vi "Create_Trajectory_Using_TrajectoryLibrary_ORIG.vi"() -> ()   [LabVIEW 2019]
doc: "This utility creates trajectories based on the robot configuration, constraints and defined waypoints."
uses:
  <vilib>/Rock Robotics/WPI/ThirdParty/JAS_Junk/TrajLib/Trajectory_Library.lvlib
  <vilib>/Utility/xml.llb/Write to XML File(string).vi
  <vilib>/Rock Robotics/WPI/ThirdParty/JAS_Junk/TrajLib/TRANSLATION2D.ctl
  <vilib>/Rock Robotics/WPI/ThirdParty/JAS_Junk/TrajLib/ROTATION2D.ctl
  <vilib>/Rock Robotics/WPI/ThirdParty/JAS_Junk/TrajLib/POSE2D.ctl
  <vilib>/Rock Robotics/WPI/ThirdParty/JAS_Junk/TrajLib/TRAJ_STATE.ctl
  <vilib>/Rock Robotics/WPI/ThirdParty/JAS_Junk/TrajLib/TRAJECTORY.ctl
  <vilib>/Utility/xml.llb/Read From XML File(string).vi
  <vilib>/Rock Robotics/WPI/ThirdParty/JAS_Junk/TrajLib/DISPLAY_WEIGHTED_WAYPOINT.ctl
  <vilib>/Rock Robotics/WPI/ThirdParty/JAS_Junk/TrajLib/DIFF_DRIVE_KINEMATICS.ctl
  <vilib>/Rock Robotics/WPI/ThirdParty/JAS_Junk/TrajLib/TRAJ_CONSTRAINT_DIIF_DRIVE_KINEMATICS.ctl
  <vilib>/Rock Robotics/WPI/ThirdParty/JAS_Junk/TrajLib/TRAJ_CONSTRAINT_CENTRIPETAL_ACCEL.ctl
  <vilib>/Analysis/Matrix/Datatypes/RealMatrix.ctl
  <vilib>/Analysis/Matrix/NI_Matrix.lvlib
  <vilib>/Rock Robotics/WPI/ThirdParty/JAS_Junk/TrajLib/SWERVE_DRIVE_KINEMATICS.ctl
  <vilib>/Rock Robotics/WPI/ThirdParty/JAS_Junk/TrajLib/TRAJ_CONSTRAINT_SWERVE_DRIVE_KINEMATICS.ctl
  <vilib>/Rock Robotics/WPI/ThirdParty/JAS_Junk/TrajLib/SIMPLE_MOTOR_FF.ctl
  <vilib>/Rock Robotics/WPI/ThirdParty/JAS_Junk/TrajLib/TRAJ_CONSTRAINT_DIIF_DRIVE_VOLTAGE.ctl
  <vilib>/Rock Robotics/WPI/ThirdParty/JAS_Junk/TrajLib/MECA_DRIVE_KINEMATICS.ctl
  <vilib>/Rock Robotics/WPI/ThirdParty/JAS_Junk/TrajLib/TRAJ_CONSTRAINT_MECA_DRIVE_KINEMATICS.ctl
  <vilib>/Rock Robotics/WPI/ThirdParty/JAS_Junk/TrajLib/TRAJ_CONFIG.ctl
  TrajCreateUnitsENUM.ctl
  TrajCreateConfig_V3.ctl
panel:
  in  "End Program":bool
  in  "Tab Control":T1(tab)
  out "Config File Read\nWithout Error":bool
  out "Config File  Read Error":errorcluster
  out "Read Config File Comment":string
  in  "Read Config File Name":path
  in  "ReadConfigFile":bool
  in  "Field Selector":string(combo)
  in  "Units Selector":T2
  in  "MaxVelocity":dbl=50.0 format="%17.1f"
  in  "MaxAcceleration":dbl=40.0 format="%17.1f"
  out "MaxVelocity M/S":dbl=2.0 format="%17.4f"
  out "MaxAcceleration M/S^2":dbl=1.3 format="%17.4f"
  in  "Right Rear":T3={"X"=-0.5, "Y"=0.5} {"Y" format="%14.3f"; "X" format="%14.3f"}
  in  "Left Rear":T3={"X"=-0.5, "Y"=-0.5} {"Y" format="%14.3f"; "X" format="%14.3f"}
  in  "Right Front":T3={"X"=0.5, "Y"=0.5} {"Y" format="%14.3f"; "X" format="%14.3f"}
  in  "Left Front":T3={"X"=0.5, "Y"=-0.5} {"Y" format="%14.3f"; "X" format="%14.3f"}
  in  "Use Centripetal\nAcceleration\nConstaint":bool=TRUE
  out "Max Cent Accel M/S^2":dbl=1.0 format="%20.4f"
  in  "Max Cent Accel":dbl=20.0 format="%20.1f"
  in  "Use Diff Drive\nKinematic\nConstraint":bool=TRUE
  out "Wheelbase Width M":dbl=0.66 format="%20.4f"
  in  "Wheelbase Width":dbl=20.866 format="%20.1f"
  in  "Max Voltage":dbl=12.0 format="%20.4f"
  in  "SIMPLE_MOTOR_FF":T4={"Ks"=0.9, "Kv"=0.22199, "Ka"=0.04876} {"Ka" format="%13.4f"; "Kv" format="%13.4f"; "Ks" format="%13.4f"}
  in  "Use Diff Drive\nVoltage\nConstraint":bool=TRUE
  in  "Wheels":T3[](array[typedef])=[{"X"=0.5, "Y"=-0.5}, {"X"=0.5, "Y"=0.5}, {"X"=-0.5, "Y"=0.5}, {"X"=-0.5, "Y"=-0.5}] {"Y" format="%14.3f"; "X" format="%14.3f"}
  in  "Use Swerve Drive\nKinematics\nConstraint":bool
  in  "Use Mecanum \nDrive Kinematics\nConstraint":bool
  out "Left Front M":T3 {"Y" format="%14.3f"; "X" format="%14.3f"}
  out "Right Front M":T3 {"Y" format="%14.3f"; "X" format="%14.3f"}
  out "Left Rear M":T3 {"Y" format="%14.3f"; "X" format="%14.3f"}
  out "Right Rear M":T3 {"Y" format="%14.3f"; "X" format="%14.3f"}
  out "SIMPLE_MOTOR_FF M":T4 {"Ka" format="%13.4f"; "Kv" format="%13.4f"; "Ks" format="%13.4f"}
  out "Wheels M":T3[](array[typedef]) {"Y" format="%14.3f"; "X" format="%14.3f"}
  in  "WayPoints":T5[](array[typedef])=[{"X"=15.0, "Y"=105.0, "ANGLE"=-45.0, "WEIGHT"=12.0}, {"X"=105.0, "Y"=65.0, "ANGLE"=0.0, "WEIGHT"=12.0}, {"X"=210.0, "Y"=106.0, "ANGLE"=45.0, "WEIGHT"=12.0}, {"X"=350.0, "Y"=105.0, "ANGLE"=-45.0, "WEIGHT"=12.0}] {"WEIGHT" format="%13.3f"; "ANGLE" format="%13.3f"; "Y" format="%13.3f"; "X" format="%13.3f"}
  in  "Spline Type":enum32{"Radio Selection 1", "Radio Selection 2"}(radio)
  in  "Reverse":bool
  in  "UseWeights":bool
  in  "Calculate\nTrajectory":bool
  out "Trajectory\nCompleted\nError Free":bool
  out "Trajectory calculation error":errorcluster
  out "Position":cluster{dbl[], dbl[]}[](graph)
  out "Field Display":T6(plugin-control)
  out "Trajectory Data":cluster{dbl[], dbl[]}[](graph)
  out "differential \ndrive \nmax speed":dbl format="%15.1f"
  out "Traj States\nSize":i32
  out "Trajectory States":T7[](array[typedef]) {"POSE"."ROTATION"."SIN" format="%13.4f"; "POSE"."ROTATION"."COS" format="%13.4f"; "POSE"."ROTATION"."VALUE" format="%13.4f"; "POSE"."TRANSLATION"."Y" format="%14.3f"; "POSE"."TRANSLATION"."X" format="%14.3f"}
  in  "Trajectory JSON File Name":path
  out "JSON File Saved\nWithout Error":bool
  out "Write CSV File Error":errorcluster
  in  "PathWeaver Length Units":T10(radio)
  in  "WriteJSONFile":bool
  out "CSV File Saved\nWithout Error":bool
  in  "Trajectory Type":enum32{"Radio Selection 1", "Radio Selection 2"}(radio)
  out "Write Trajectory\nFile Error":errorcluster
  in  "Trajectory File Comment":string
  in  "Trajectory CSV File Name":path
  in  "WriteTrajFile":bool
  out "Config File Saved\nWithout Error":bool
  out "Write Config FIle Error":errorcluster
  in  "Write Config File Comment":string
  in  "Write Config File Name":path
  in  "WriteConfigFile":bool
  # "Create Trajectory  (Use LabVIEW trajectory library)"
  # "Instructions:  \n----------------\n\nThis utility will create a trajectory, show the data on the various tabs, and optionally write a \"field absolute\" or \"robot relative\" trajectory to a file. \nTo use this utility:\n\n1) Read all of these instructions!\n2) Define the robot's physical data on the \"Robot Data\" tab.  \n3) Define the robot's movement constraints on the \"Constraints\" page.  \n4) Define the trajectory on the \"Define/Create Trajectory\" tab.  These are the beginning and ending positions/headings, and internal positions/headings.  \n    Cubic splines only use the first and last \"angle\".  The other internal \"angles\" are calculated.  Quintic splines use all the defined angles.\n5) Press the \"Calculate Trajectory\".  If a good trajectory was calculated it will be displayed.  If no errors are generated the Trajectory Complete\n    light will be on.  Errors will be displayed in the error indicator.  The path can be recalculated many times before performing any other action.\n\nAfter a Trajectory has been calculated, the \"trajectory can be written to a file.  The absolute path is converted to a robot relative trajectory.  To do this:\n1) Enter a comment to be included in the file.  Anything can be entered.\n2) Select the file name.\n3) Press \"Create Trajectory File\"  If an error occurs it will be displayed in the File Creation Error indicator.\n\nNotes:\n--------\n- All the robot parameters, path, and field dimensions are in UNITS, and DEGREES.  Select UNITS from the \"Robot Data\" page.  The resulting  \n  trajectory is converted to METERS, and RADIANS to match the rest of this library!\n- The trajectory library is the same as the WPILIB spline and trajectory library for Java and C++.\n- 2019 playing field size - width: 26 ft 11.25 In = 323.25 in , length: 52 ft 5.25 in = 629.25 in  (I didn't verify this for the 2020 version.)"
  # "Read Trajectory Waypoints and Configuration from File"
  # "ROBOT DATA"
  # "UNITS/SEC"
  # "Meters/SEC"
  # "UNITS/SEC^2"
  # "Meters/SEC^2"
  # "Simulated robot max speed is: 68.266 Inches/Second"
  # "UTILITY CONFIGURATION"
  # "Diff Kinematics Constraint"
  # "Centripetal Accel Constraint"
  # "Diff Voltage Constraint"
  # "UNITS"
  # "UNITS/SEC^2"
  # "VOLTS"
  # "METERS"
  # "METERS/SEC^2"
  # "Distance is:\nUNITS"
  # "Simulated robot wheelbase is 20.87 in"
  # "Ks = Volts\nKv = VoltSec/Meter\nKa = Volt(Sec^2)/Meter"
  # "Swerve Kinematics Constraint"
  # "Mechanum Kinematics Constraint"
  # "Values\nare \nUNITS"
  # "Values\nare \nUNITS"
  # "TRAJECTORY DEFINITION"
  # "To delete array elements or the entire array, right click on the array or element, select Data Operations, then select the action to be performed."
  # "UNITS, UNITS, DEGREES, SCALAR"
  # "INCHES/SEC"
  # "Write Trajectory to File   -   CSV, and / or JSON"
  # "Write Trajectory Waypoints and Configuration to File"
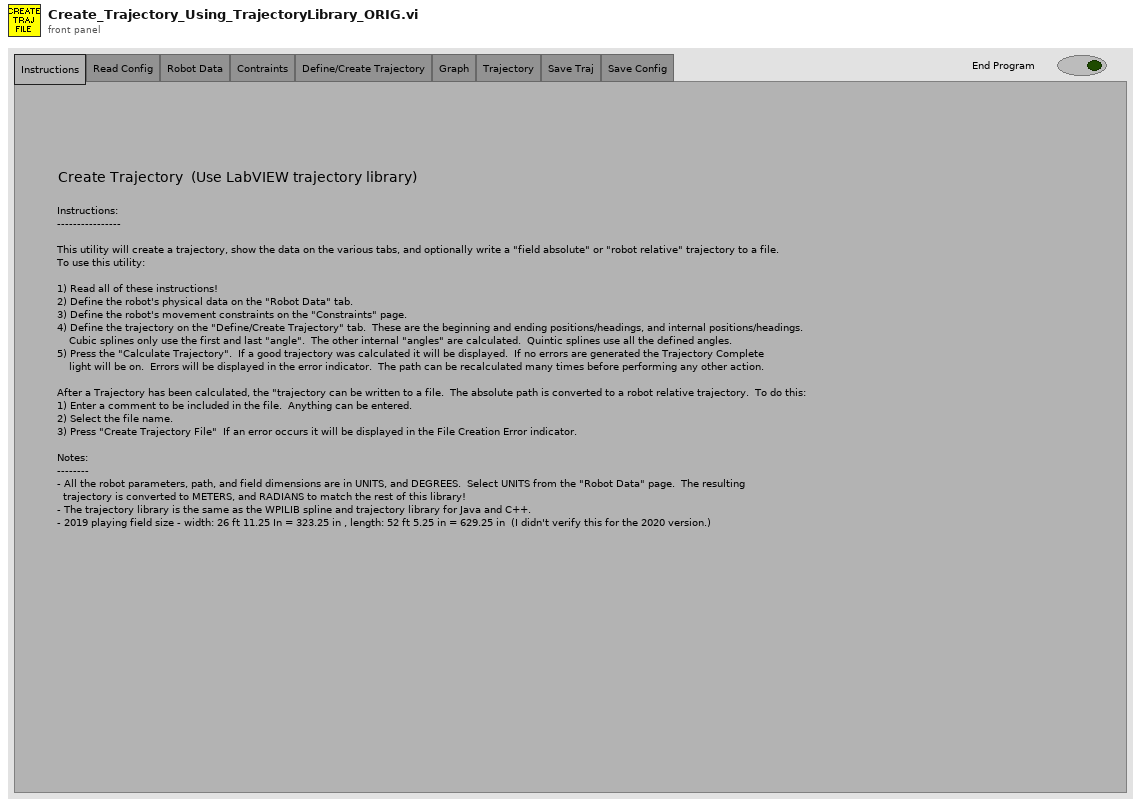
[diagram p1: front panel]
types:
  T1 = enum32{"Instructions", "Read Config", "Robot Data", "Contraints", "Define/Create Trajectory", "Graph", "Trajectory", "Save Traj", "Save Config"}
  T2 = typedef "TrajCreateUnitsENUM.ctl" = enum16{"Inches", "Feet", "Centimeters", "Meters"}
  T3 = typedef "Trajectory_Library.lvlib/TRANSLATION2D.ctl" = cluster{"X":dbl, "Y":dbl}
  T4 = typedef "Trajectory_Library.lvlib/SIMPLE_MOTOR_FF.ctl" = cluster{"Ks":dbl, "Kv":dbl, "Ka":dbl}
  T5 = typedef "Trajectory_Library.lvlib/DISPLAY_WEIGHTED_WAYPOINT.ctl" = cluster{"X":dbl, "Y":dbl, "ANGLE":dbl, "WEIGHT":dbl}
  T6 = typedef "IMAQ Image.ctl" = refnum<image>
  T7 = typedef "Trajectory_Library.lvlib/TRAJ_STATE.ctl" = cluster{"TimeSeconds":dbl, "Velocity":dbl, "Acceleration":dbl, "POSE":T8, "Curvature":dbl}
  T8 = typedef "Trajectory_Library.lvlib/POSE2D.ctl" = cluster{"TRANSLATION":T3, "ROTATION":T9}
  T9 = typedef "Trajectory_Library.lvlib/ROTATION2D.ctl" = cluster{"VALUE":dbl, "COS":dbl, "SIN":dbl}
  T10 = enum32{"Radio Selection 1", "Radio Selection 2", "Radio Selection 3", "Radio Selection 4", "Radio Selection 5"}
  T11 = typedef "Image Type" = u32
  T12 = enum8{"Enabled", "Disabled", "Disabled and Grayed Out"}
  T13 = typedef "Trajectory_Library.lvlib/TRAJECTORY.ctl" = cluster{"TotalTImeSecs":dbl, "States":T7[]}
  T14 = typedef "TrajCreateConfig_V3.ctl" = cluster{"Write Config File Name":path, "Write Config File Comment":string, "WayPoints":T5[], "TRAJECTORY_CONFIG":T15, "IsCubic":bool, "Units Selector":T2, "UseWeights":bool}
  T15 = typedef "Trajectory_Library.lvlib/TRAJ_CONFIG.ctl" = cluster{"MaxVelocity":dbl, "Max Acceleration":dbl, "StartVelocity":dbl, "End Velocity":dbl, "Reversed":bool, "DiffDrKineConstntDefined":bool, "CentAcellConstntDefined":bool, "DiffDrVoltConstntDefined":bool, "DIFF_DRIVE_KINE_CONSTRAINT":T16, "CENTRIPETAL_ACCEL_CONSTRAINT":T18, "SwerveDrKineConstntDefined":bool, "SWERVE_DRIVE_KINE_CONSTRAINT":T19, "DIFF_DRIVE_VOLTAGE_CONSTRAINT":T22, "MECANUM_DRIVE_KINE_CONSTRAINT":T23, "MecanumDrKineConstntDefined":bool}
  T16 = typedef "Trajectory_Library.lvlib/TRAJ_CONSTRAINT_DIIF_DRIVE_KINEMATICS.ctl" = cluster{"Max Speed (M/S)":dbl, "DIFF_DRIVE_KINEMATICS":T17, "Max Accel (M/S2)":dbl}
  T17 = typedef "Trajectory_Library.lvlib/DIFF_DRIVE_KINEMATICS.ctl" = cluster{"TrackWidth_Meters":dbl}
  T18 = typedef "Trajectory_Library.lvlib/TRAJ_CONSTRAINT_CENTRIPETAL_ACCEL.ctl" = cluster{"Max Cent Accel":dbl}
  T19 = typedef "Trajectory_Library.lvlib/TRAJ_CONSTRAINT_SWERVE_DRIVE_KINEMATICS.ctl" = cluster{"Max Speed (M/S)":dbl, "SwerveKinematics":T20}
  T20 = typedef "Trajectory_Library.lvlib/SWERVE_DRIVE_KINEMATICS.ctl" = cluster{"NumModules":i32, "InverseKinematics":T21, "ForwardKinematics":T21, "Modules":T3[], "PrevCoR":T3}
  T21 = typedef "NI_Matrix.lvlib/RealMatrix.ctl" = dbl[][]
  T22 = typedef "Trajectory_Library.lvlib/TRAJ_CONSTRAINT_DIIF_DRIVE_VOLTAGE.ctl" = cluster{"Max Voltage":dbl, "DIFF_DRIVE_KINEMATICS":T17, "SIMPLE_MOTOR_FF":T4}
  T23 = typedef "Trajectory_Library.lvlib/TRAJ_CONSTRAINT_MECA_DRIVE_KINEMATICS.ctl" = cluster{"Max Speed (M/S)":dbl, "MECA_DRIVE_KINEMATICS":T24}
  T24 = typedef "Trajectory_Library.lvlib/MECA_DRIVE_KINEMATICS.ctl" = cluster{"FrontLeft":T3, "FrontRight":T3, "RearLeft":T3, "RearRight":T3, "InverseKinematics":T21, "ForwardKinematics":T21, "PrevCoR":T3}
  T25 = typedef "TrajectoryUtils_Field_Info.ctl" = cluster{"FIeld_File_Name":string, "Top_Left_X":i32, "Top_Left_Y":i32, "Bottom_Right_X":i32, "Bottom_Right_Y":i32, "Field_Size_X":dbl, "Field_Size_Y":dbl, "FIeld_Size_Units":string}
  T26 = typedef "Trajectory_Library.lvlib/WEIGHTED_WAYPOINT.ctl" = cluster{"TRANSLATION":T3, "ROTATION":T9, "SCALAR":dbl}
  T27 = typedef "Trajectory_Library.lvlib/SPLINE_CTRL_VECTOR.ctl" = cluster{"Xs":dbl[], "Ys":dbl[]}
  T28 = typedef "Trajectory_Library.lvlib/CHASSIS_SPEEDS.ctl" = cluster{"vX":dbl, "vY":dbl, "vOmega":dbl}
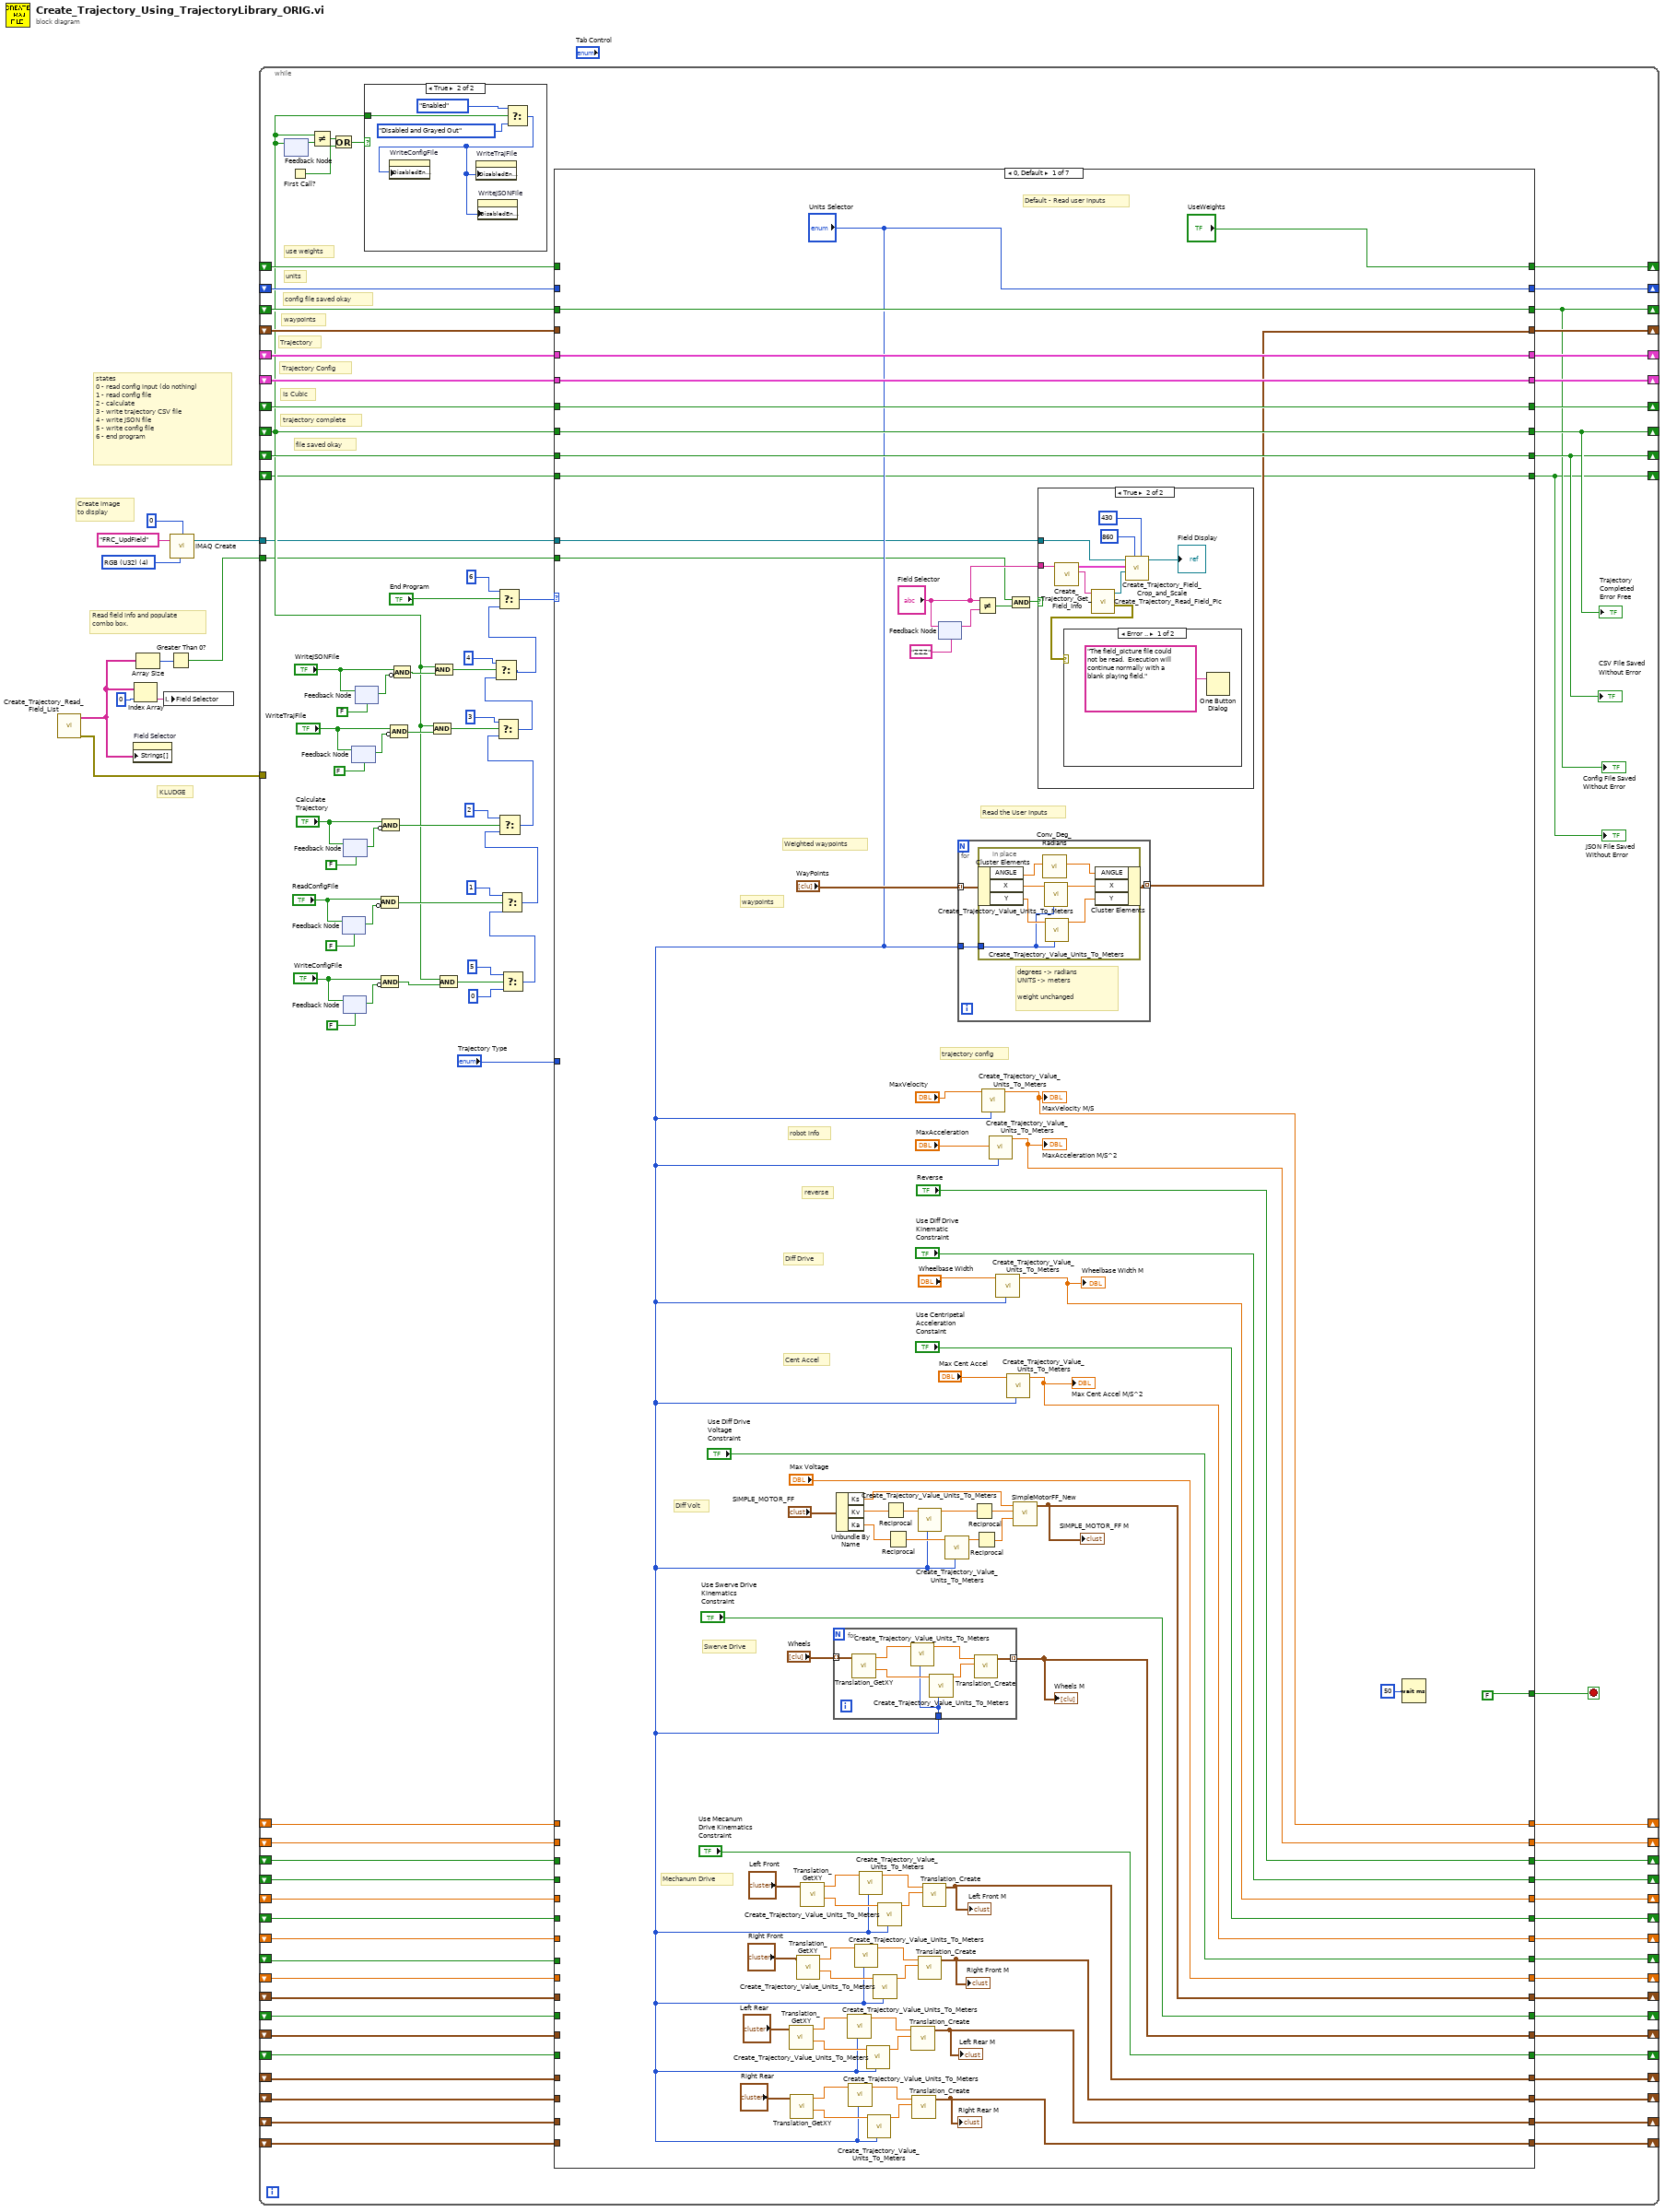
[diagram p0: block diagram]
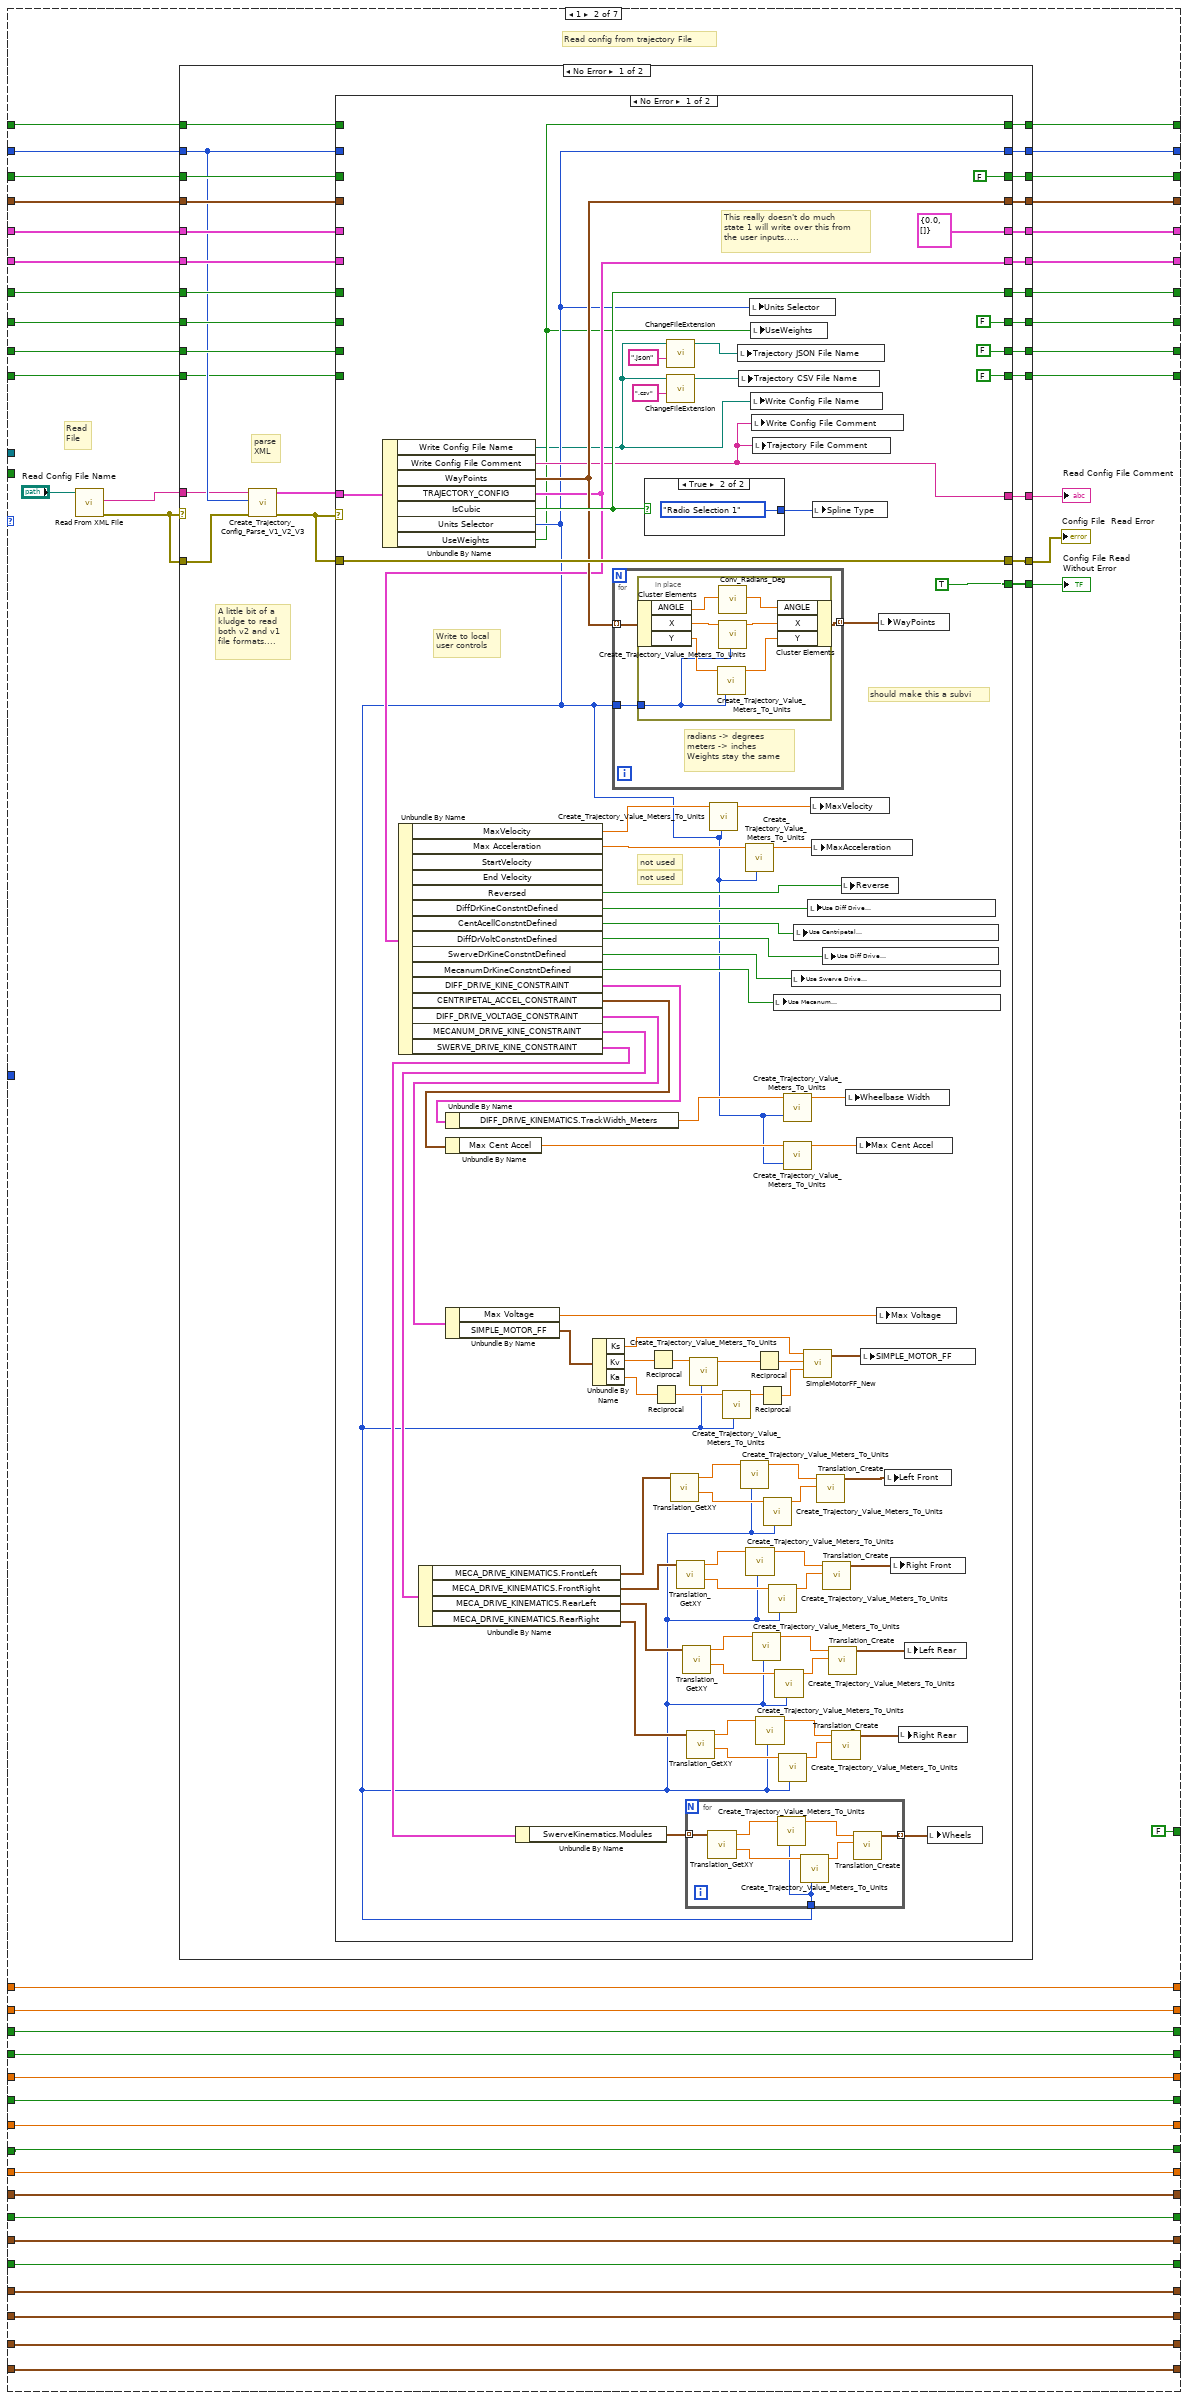
[diagram p5: hidden frame]
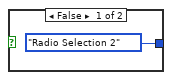
[diagram p6: hidden frame]
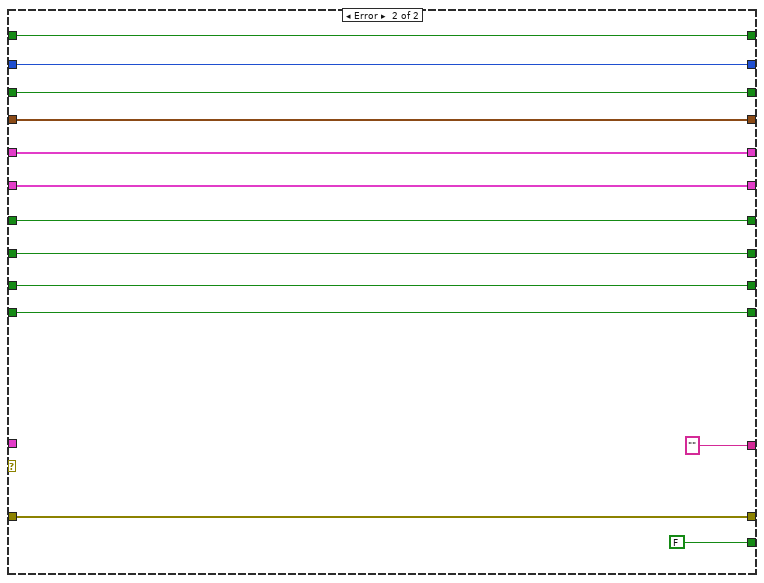
[diagram p7: hidden frame]
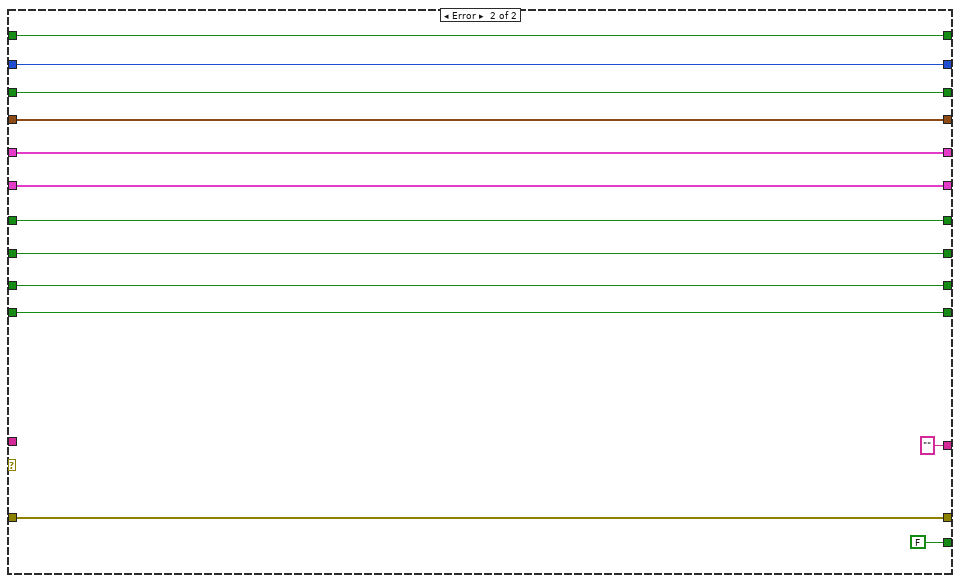
[diagram p8: hidden frame]
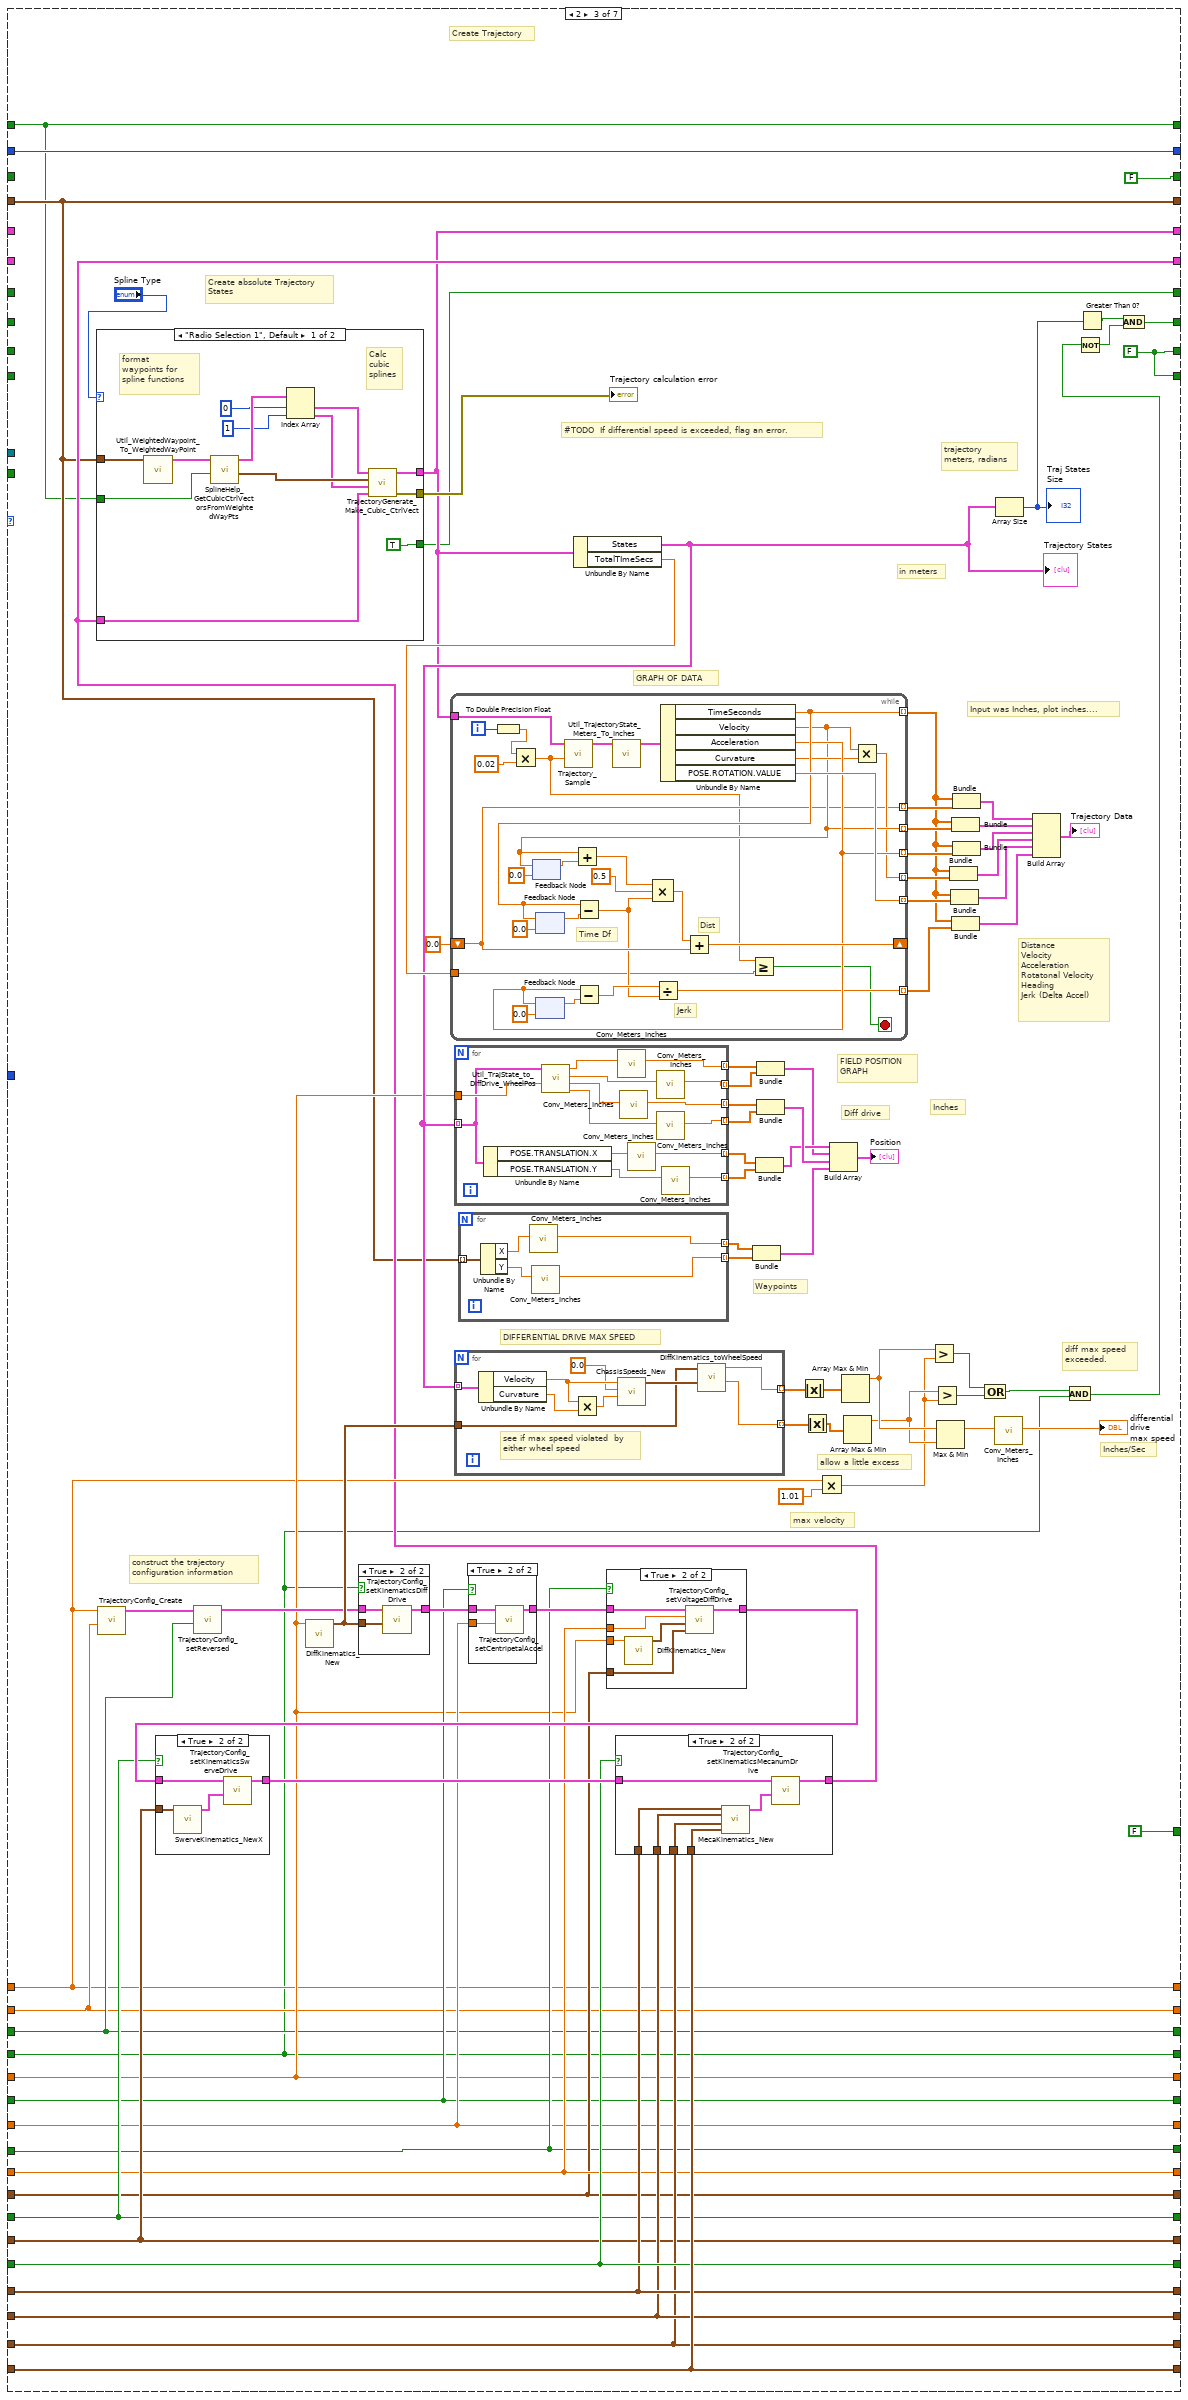
[diagram p9: hidden frame]
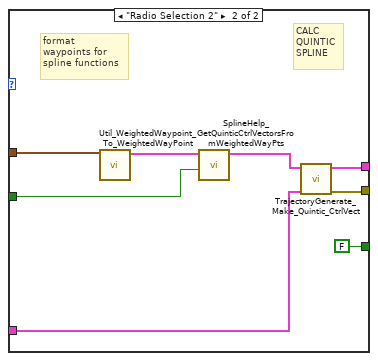
[diagram p13: hidden frame]
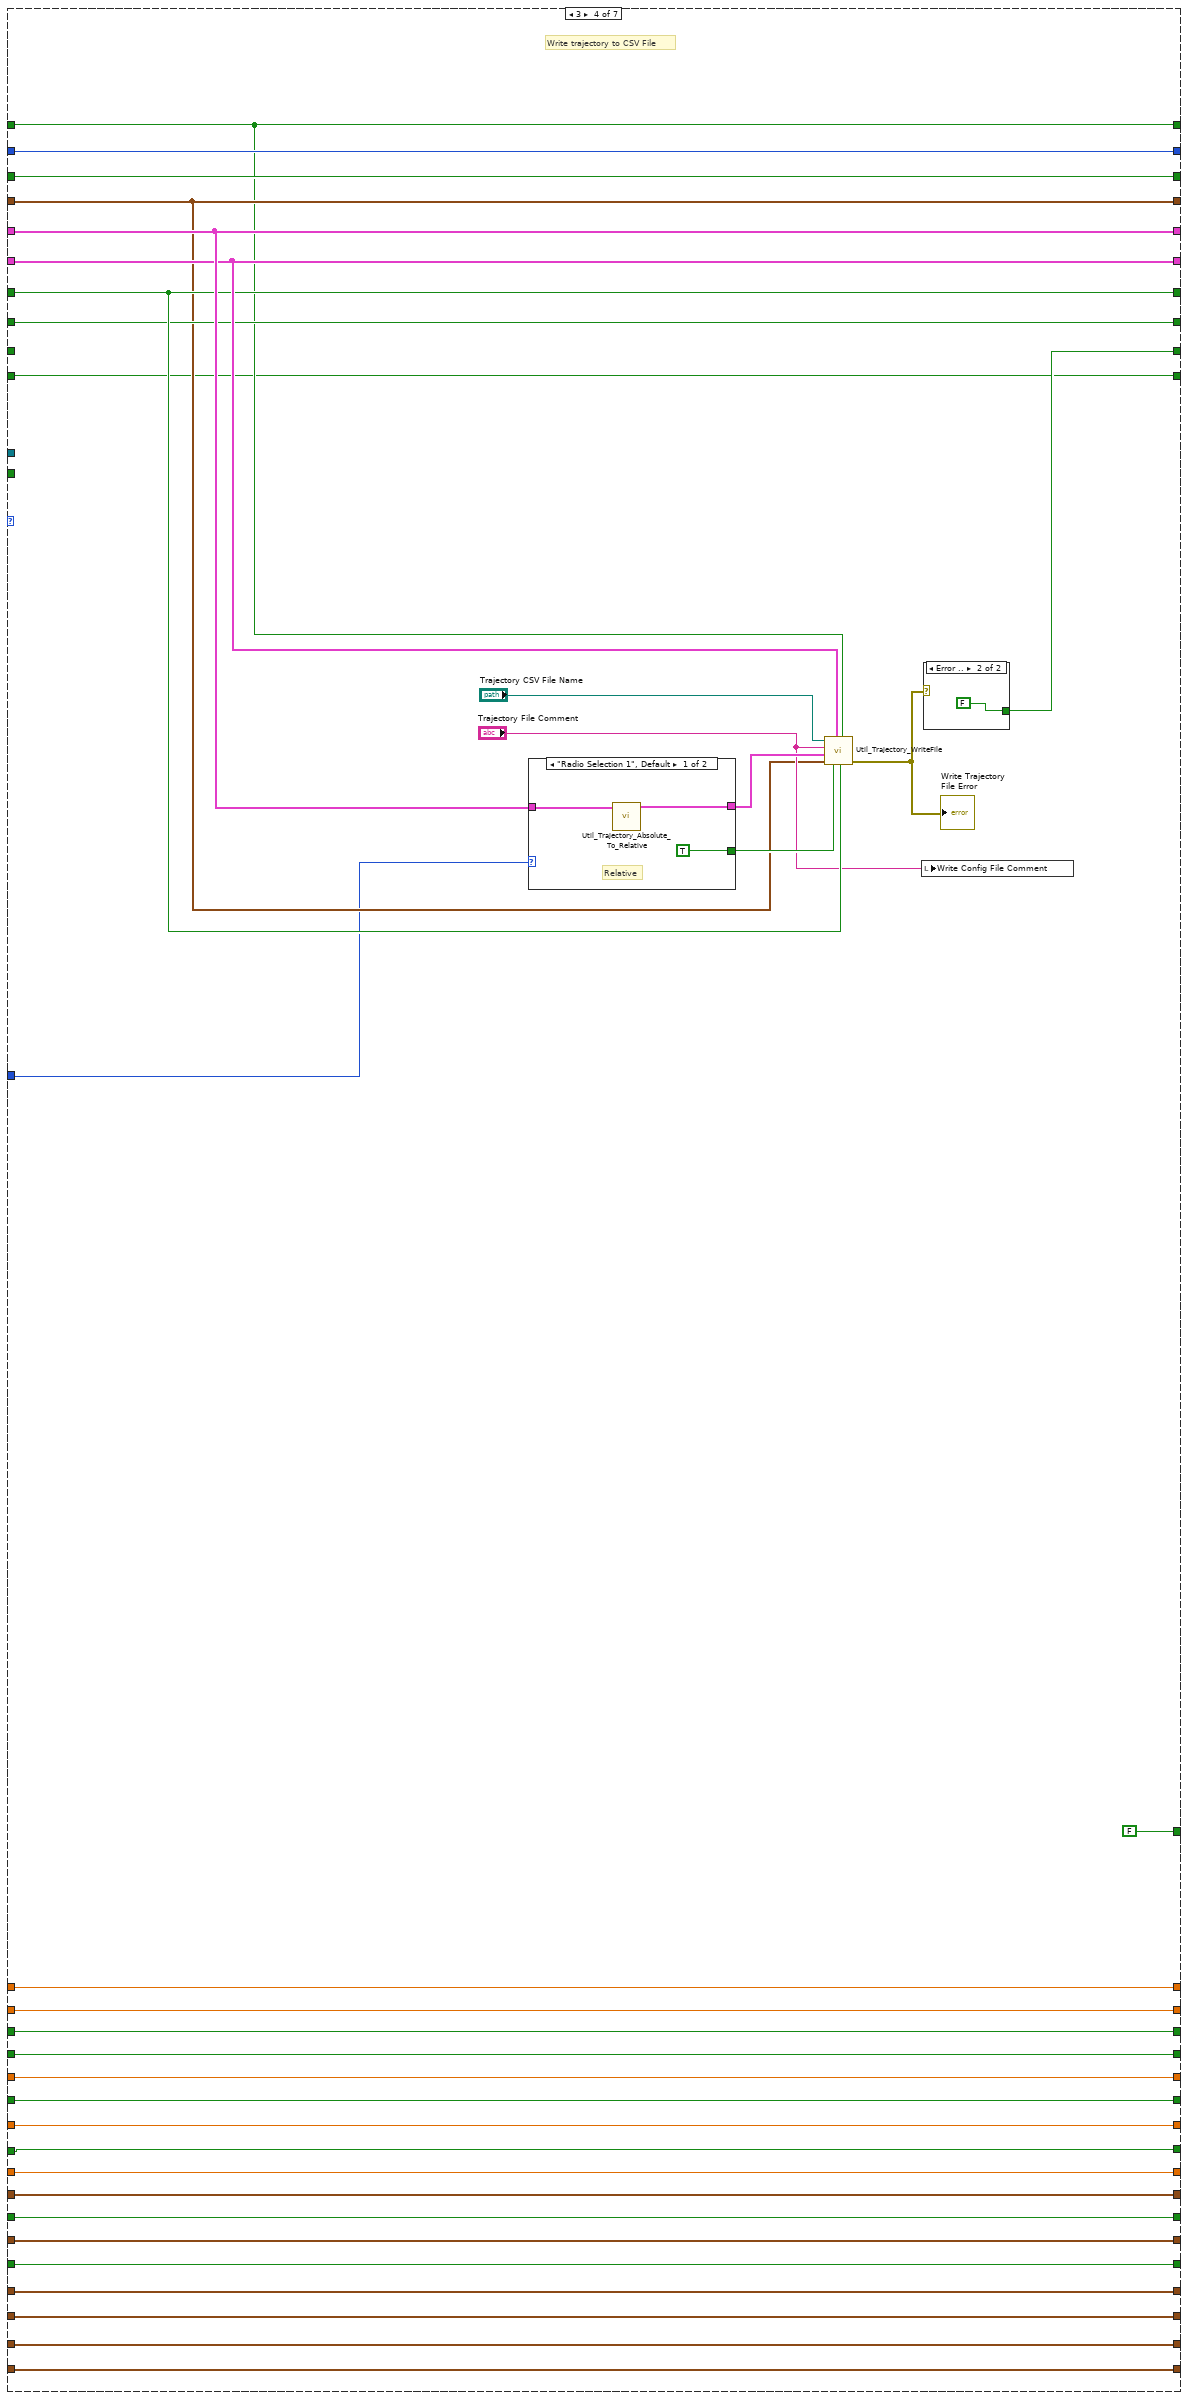
[diagram p16: hidden frame]
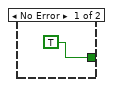
[diagram p17: hidden frame]
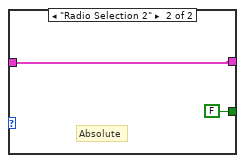
[diagram p18: hidden frame]
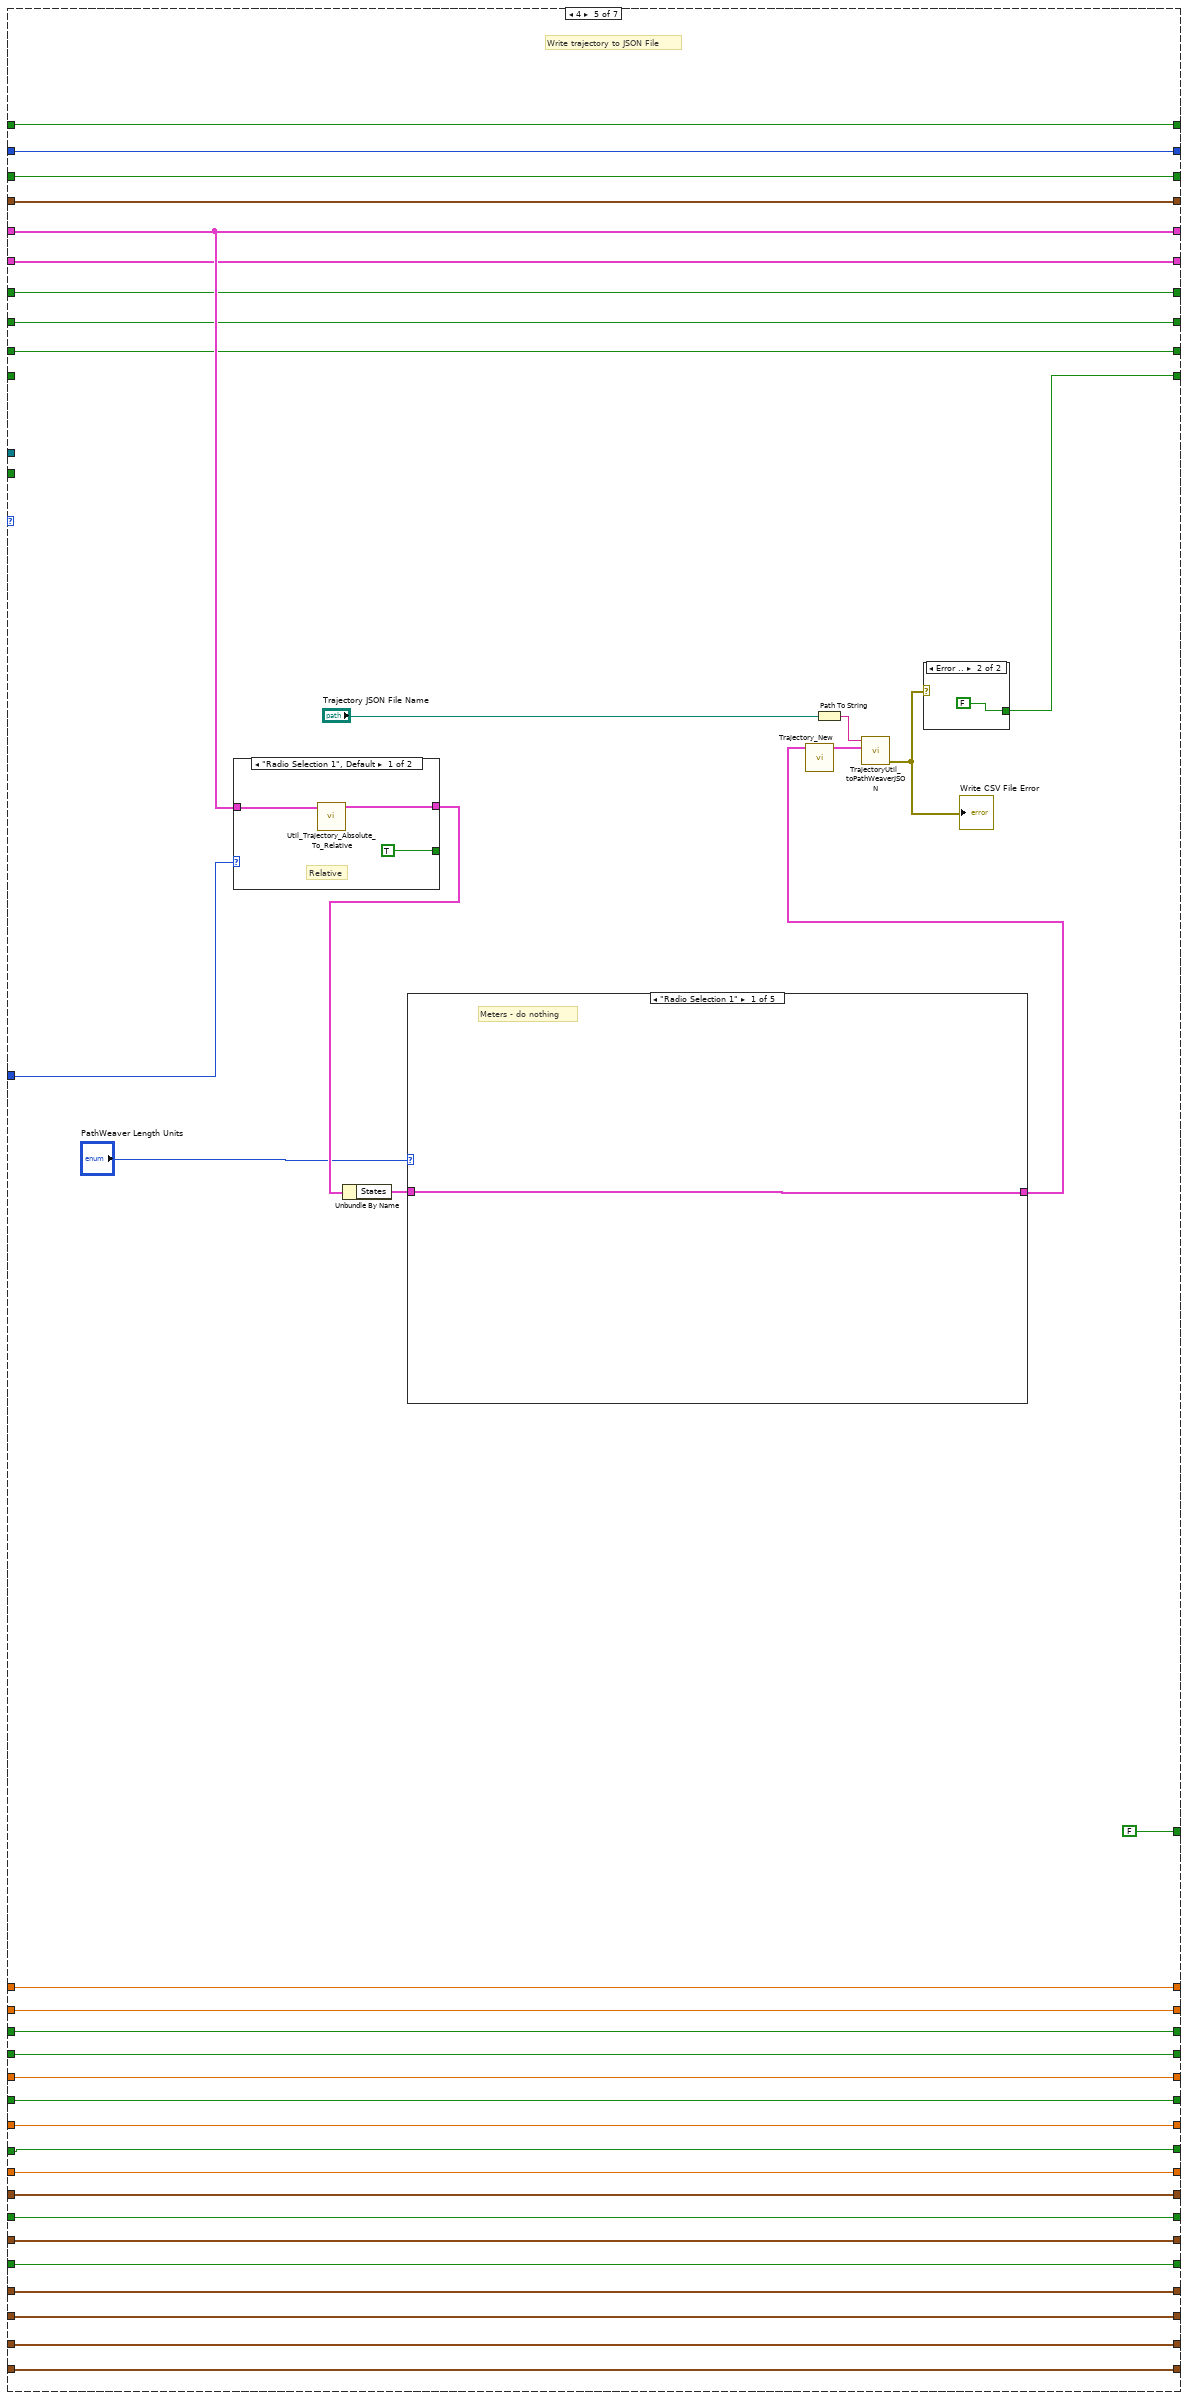
[diagram p19: hidden frame]
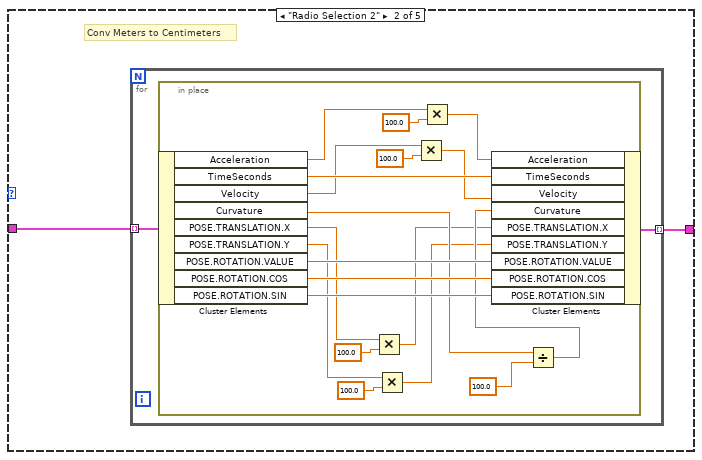
[diagram p20: hidden frame]
diagram:
  w5 = T11 4 items=["Grayscale (U8)", "Grayscale (I16)", "Grayscale (SGL)", "Complex (CSG)", "RGB (U32)", "HSL (U32)", "RGB (U64)", "Grayscale (U16)"] ("Image Type")
  # "Create image \nto display"
  # "KLUDGE"
  # "Read field info and populate\ncombo box."
  # "states\n0 - read config input (do nothing)\n1 - read config file\n2 - calculate\n3 - write trajectory CSV file\n4 - write JSON file\n5 - write config file\n6 - end program"
  n1 = call "Create_Trajectory_Read_Field_List.vi"() -> ("error out"=w8:errorcluster, "section names"=w3:string[])  [unwired: 10 in]
  n2 = property on="Field Selector" class="CmbBox"("Strings[]"=w3) -> ()  [unwired: 2 in, 2 out]
  n3 = Index Array(array=w3, index=0) -> (element=w9:string)
  n4 = Array Size(array=w3) -> (size(s)=w2:i32)
  n5 = local write "Field Selector"(w9) -> ()
  n6 = Greater Than 0?(x=w2) -> (x > 0?=w1:bool)
  n7 = call "IMAQ Create"("Border Size"=0, "Image Name"="FRC_UpdField", "Image Type"=w5) -> ("New Image"=w4:T6)  [unwired: 2 in, 1 out]
  n8 = while {
    shift-right: [w100] -> _
    shift-left: _ -> [w99]
    shift-right: [w98] -> _
    shift-left: _ -> [w97]
    shift-right: [w82] -> _
    shift-left: _ -> [w83]
    shift-right: [w85] -> _
    shift-left: _ -> [w84]
    shift-right: [w81] -> _
    shift-left: _ -> [w20]
    shift-right: [w77] -> _
    shift-left: _ -> [w78]
    shift-right: [w67] -> _
    shift-left: _ -> [w72]
    shift-right: [w76] -> _
    shift-left: _ -> [w71]
    shift-right: [w68] -> _
    shift-left: _ -> [w75]
    shift-right: [w69] -> _
    shift-left: _ -> [w74]
    shift-right: [w70] -> _
    shift-left: _ -> [w73]
    shift-right: [w66] -> _
    shift-left: _ -> [w64]
    shift-right: [w65] -> _
    shift-left: _ -> [w63]
    shift-right: [w60] -> _
    shift-left: _ -> [w61]
    shift-right: [w59] -> _
    shift-left: _ -> [w62]
    shift-right: [w57] -> _
    shift-left: _ -> [w58]
    shift-right: [w53] -> _
    shift-left: _ -> [w55]
    shift-right: [w54] -> _
    shift-left: _ -> [w56]
    shift-right: [w50] -> _
    shift-left: _ -> [w52]
    shift-right: [w49] -> _
    shift-left: _ -> [w51]
    shift-right: [w43] -> _
    shift-left: _ -> [w46]
    shift-right: [w44] -> _
    shift-left: _ -> [w47]
    shift-right: [w45] -> _
    shift-left: _ -> [w48]
    shift-right: [w30] -> _
    shift-left: _ -> [w29]
    shift-right: [w28] -> _
    shift-left: _ -> [w27]
    shift-right: [w26] -> _
    shift-left: _ -> [w25]
    shift-right: [w15] -> _
    shift-left: _ -> [w14]
    tunnel: w8 -> [_]
    tunnel: w4 -> [w12]
    tunnel: w1 -> [w11]
    stop <- w79 stop-if-true
    # "use weights"
    # "units"
    # "config file saved okay"
    # "file saved okay"
    # "trajectory complete"
    # "Is Cubic"
    # "waypoints"
    # "Trajectory Config"
    # "Trajectory"
    n9 = feedback-in #1(w20) -> ()
    n10 = feedback #1() -> (w34:bool)  [unwired: 1 in]
    n11 = First Call?() -> (First Call?: T/F=w32:bool)
    n12 = Not Equal?(x=w20, y=w34) -> (x != y?=w33:bool)
    n13 = Or(x=w33, y=w32) -> (x .or. y?=w31:bool)
    n14 = feedback #2(FALSE ("CreateCmdList")) -> (w103:bool)
    n15 = feedback-in #2("ReadConfigFile") -> ()
    n16 = feedback #3(FALSE ("CreateCmdList")) -> (w42:bool)
    n17 = feedback-in #3("WriteConfigFile") -> ()
    n18 = feedback #4(FALSE ("CreateCmdList")) -> (w106:bool)
    n19 = feedback-in #4("Calculate\nTrajectory") -> ()
    n20 = feedback-in #5("WriteTrajFile") -> ()
    n21 = feedback #5(FALSE ("CreateCmdList")) -> (w108:bool)
    n22 = feedback #6(FALSE ("CreateCmdList")) -> (w24:bool)
    n23 = feedback-in #6("WriteJSONFile") -> ()
    n24 = case shown="True" w31 {
      tunnel: w20 -> [_ w113]
      frame False {
      }
      frame True {
        n25 = Select(t=T12."Enabled" ("Disabled"), s=w113, f=T12."Disabled and Grayed Out" ("Disabled")) -> (s? t:f=w110:T12)
        n26 = property on="WriteConfigFile" class="Bool"("DisabledEnum"=w110) -> ()  [unwired: 2 in, 2 out]
        n27 = property on="WriteTrajFile" class="Bool"("DisabledEnum"=w110) -> ()  [unwired: 2 in, 2 out]
        n28 = property on="WriteJSONFile" class="Bool"("DisabledEnum"=w110) -> ()  [unwired: 2 in, 2 out]
      }
    }
    n29 = Compound Arithmetic op=AND("ReadConfigFile", invert w103) -> (w87:bool)
    n30 = Compound Arithmetic op=AND("WriteConfigFile", invert w42) -> (w35:bool)
    n31 = Compound Arithmetic op=AND("Calculate\nTrajectory", invert w106) -> (w90:bool)
    n32 = Compound Arithmetic op=AND("WriteTrajFile", invert w108) -> (w80:bool)
    n33 = Compound Arithmetic op=AND("WriteJSONFile", invert w24) -> (w21:bool)
    n34 = And(x=w20, y=w80) -> (x .and. y?=w93:bool)
    n35 = And(x=w20, y=w21) -> (x .and. y?=w18:bool)
    n36 = And(x=w20, y=w35) -> (x .and. y?=w36:bool)
    n37 = Select(t=5, s=w36, f=0) -> (s? t:f=w38:i32)
    n38 = Select(t=1, s=w87, f=w38) -> (s? t:f=w88:i32)
    n39 = Select(t=2, s=w90, f=w88) -> (s? t:f=w91:i32)
    n40 = Select(t=3, s=w93, f=w91) -> (s? t:f=w17:i32)
    n41 = Select(t=4, s=w18, f=w17) -> (s? t:f=w16:i32)
    n42 = Select(t=6, s="End Program", f=w16) -> (s? t:f=w86:i32)
    n43 = case shown="0, Default" w86 {
      tunnel: w52 -> [_ w251 w425 w607 w656 w794 w828]
      tunnel: w56 -> [_ w249 w427 w609 w658 w796 w826]
      tunnel: w51 -> [_ w252 w416 w606 w655 w793 w829]
      tunnel: w55 -> [_ w250 w426 w608 w657 w795 w827]
      tunnel: w58 -> [_ w248 w428 w610 w659 w797 w825]
      tunnel: w62 -> [_ w246 w429 w612 w661 w799 w823]
      tunnel: w61 -> [_ w247 w430 w611 w660 w798 w824]
      tunnel: w63 -> [_ w245 w431 w613 w662 w800 w822]
      tunnel: w64 -> [_ w244 w432 w614 w663 w801 w821]
      tunnel: w73 -> [_ w243 w436 w615 w664 w802 w820]
      tunnel: w74 -> [_ w242 w435 w616 w665 w803 w819]
      tunnel: w75 -> [_ w241 w434 w617 w666 w804 w818]
      tunnel: w71 -> [_ w239 w437 w619 w668 w806 w816]
      tunnel: [w185 w229 w420 w624 w672 w808 w837] -> w100
      tunnel: w99 -> [w185 w235 _ w624 w672 w808 w837]
      tunnel: [w184 w228 w421 w623 w671 w788 w836] -> w98
      tunnel: w97 -> [w184 w234 _ w623 w671 w788 w836]
      tunnel: [w183 w227 w419 w622 w670 w787 w835] -> w82
      tunnel: [w124 w230 w413 w599 w649 w789 w838] -> w85
      tunnel: w84 -> [_ w236 w413 w599 w649 w789 w838]
      tunnel: w83 -> [w183 w233 _ w622 w670 w787 w835]
      tunnel: [w182 w226 w444 w621 w669 w807 w834] -> w81
      tunnel: w20 -> [w182 w232 _ w621 w669 w807 w834]
      tunnel: [FALSE FALSE FALSE FALSE FALSE FALSE TRUE] -> w79
      tunnel: [w179 w225 w407 w620 w646 w786 w833] -> w77
      tunnel: w78 -> [w179 w231 _ _ w646 w786 w833]
      tunnel: [w139 w239 w437 w619 w668 w806 w816] -> w76
      tunnel: w72 -> [_ w240 w433 w618 w667 w805 w817]
      tunnel: ["Use Mecanum \nDrive Kinematics\nConstraint" w243 w436 w615 w664 w802 w820] -> w70
      tunnel: [w160 w242 w435 w616 w665 w803 w819] -> w69
      tunnel: [w141 w241 w434 w617 w666 w804 w818] -> w68
      tunnel: [w140 w240 w433 w618 w667 w805 w817] -> w67
      tunnel: [w126 w244 w432 w614 w663 w801 w821] -> w66
      tunnel: ["Use Swerve Drive\nKinematics\nConstraint" w245 w431 w613 w662 w800 w822] -> w65
      tunnel: ["Max Voltage" w247 w430 w611 w660 w798 w824] -> w60
      tunnel: [w138 w246 w429 w612 w661 w799 w823] -> w59
      tunnel: ["Use Diff Drive\nVoltage\nConstraint" w248 w428 w610 w659 w797 w825] -> w57
      tunnel: [w171 w249 w427 w609 w658 w796 w826] -> w54
      tunnel: ["Use Centripetal\nAcceleration\nConstaint" w250 w426 w608 w657 w795 w827] -> w53
      tunnel: [w168 w251 w425 w607 w656 w794 w828] -> w50
      tunnel: ["Use Diff Drive\nKinematic\nConstraint" w252 w416 w606 w655 w793 w829] -> w49
      tunnel: w48 -> [_ w253 w424 w605 w654 w792 w830]
      tunnel: w47 -> [_ w254 w423 w604 w653 w791 w831]
      tunnel: w46 -> [_ w255 w422 w603 w652 w790 w832]
      tunnel: ["Reverse" w253 w424 w605 w654 w792 w830] -> w45
      tunnel: [w165 w254 w423 w604 w653 w791 w831] -> w44
      tunnel: [w164 w255 w422 w603 w652 w790 w832] -> w43
      tunnel: [w163 w220 FALSE ("File Saved\nWithout\nError") w602 w651 w780 w815] -> w30
      tunnel: w29 -> [w163 w219 _ w602 w651 _ w815]
      tunnel: ["Units Selector" w217 w414 w601 w650 w778 w814] -> w28
      tunnel: w27 -> [_ w218 w414 w601 w650 w778 w814]
      tunnel: ["UseWeights" w216 w408 w598 w648 w776 w813] -> w26
      tunnel: w25 -> [_ w215 w408 w598 w648 w776 w813]
      tunnel: [w121 w214 w407 w597 w647 w775 w812] -> w15
      tunnel: w14 -> [w121 w213 _ w597 _ w775 w812]
      tunnel: "Trajectory Type" -> [_ _ _ w596 w645 _ _]
      tunnel: w12 -> [w117 _ _ _ _ _ _]
      tunnel: w11 -> [w114 _ _ _ _ _ _]
      frame 0, Default {
        # "Weighted waypoints"
        # "reverse"
        # "robot info"
        # "Diff Drive"
        # "Cent Accel"
        # "Diff Volt"
        # "Swerve Drive"
        # "Mechanum Drive"
        # "Read the User Inputs"
        # "trajectory config"
        # "waypoints"
        # "Default - Read user inputs"
        n44 = call <vilib>:"Translation_GetXY.vi"("In Translation"="Left Rear") -> ("Y"=w149:dbl, "X"=w151:dbl)  [unwired: 9 in]
        n45 = call <vilib>:"Translation_GetXY.vi"("In Translation"="Right Rear") -> ("Y"=w144:dbl, "X"=w146:dbl)  [unwired: 9 in]
        n46 = call <vilib>:"Translation_GetXY.vi"("In Translation"="Right Front") -> ("Y"=w154:dbl, "X"=w156:dbl)  [unwired: 9 in]
        n47 = call <vilib>:"Translation_GetXY.vi"("In Translation"="Left Front") -> ("Y"=w159:dbl, "X"=w162:dbl)  [unwired: 9 in]
        n48 = for {
          tunnel: "Wheels" -> [w208] mode=indexing
          tunnel: [w207] -> w126 mode=indexing
          tunnel: "Units Selector" -> [w206]
          n49 = call <vilib>:"Translation_GetXY.vi"("In Translation"=w208) -> ("Y"=w210:dbl, "X"=w212:dbl)  [unwired: 9 in]
          n50 = call "Create_Trajectory_Value_Units_To_Meters.vi"("Units Selector"=w206, "Units"=w212) -> ("Meters"=w211:dbl)  [unwired: 9 in]
          n51 = call "Create_Trajectory_Value_Units_To_Meters.vi"("Units Selector"=w206, "Units"=w210) -> ("Meters"=w209:dbl)  [unwired: 9 in]
          n52 = call <vilib>:"Translation_Create.vi"("Y"=w209, "X"=w211) -> ("TRANSLATION"=w207:T3)  [unwired: 9 in]
        }
        "Wheels M" <- w126
        n53 = Unbundle By Name("SIMPLE_MOTOR_FF") -> ("Ks"=w136:dbl, "Kv"=w135:dbl, "Ka"=w128:dbl)
        n54 = call "Create_Trajectory_Value_Units_To_Meters.vi"("Units Selector"="Units Selector", "Units"=w151) -> ("Meters"=w150:dbl)  [unwired: 9 in]
        n55 = call "Create_Trajectory_Value_Units_To_Meters.vi"("Units Selector"="Units Selector", "Units"=w146) -> ("Meters"=w145:dbl)  [unwired: 9 in]
        n56 = call "Create_Trajectory_Value_Units_To_Meters.vi"("Units Selector"="Units Selector", "Units"=w156) -> ("Meters"=w155:dbl)  [unwired: 9 in]
        n57 = call "Create_Trajectory_Value_Units_To_Meters.vi"("Units Selector"="Units Selector", "Units"=w162) -> ("Meters"=w161:dbl)  [unwired: 9 in]
        n58 = call "Create_Trajectory_Value_Units_To_Meters.vi"("Units Selector"="Units Selector", "Units"=w149) -> ("Meters"=w148:dbl)  [unwired: 9 in]
        n59 = call "Create_Trajectory_Value_Units_To_Meters.vi"("Units Selector"="Units Selector", "Units"=w144) -> ("Meters"=w143:dbl)  [unwired: 9 in]
        n60 = call "Create_Trajectory_Value_Units_To_Meters.vi"("Units Selector"="Units Selector", "Units"=w154) -> ("Meters"=w153:dbl)  [unwired: 9 in]
        n61 = call "Create_Trajectory_Value_Units_To_Meters.vi"("Units Selector"="Units Selector", "Units"=w159) -> ("Meters"=w158:dbl)  [unwired: 9 in]
        n62 = Reciprocal(x=w135) -> (1/x=w134:dbl)
        n63 = Reciprocal(x=w128) -> (1/x=w131:dbl)
        n64 = call <vilib>:"Translation_Create.vi"("Y"=w148, "X"=w150) -> ("TRANSLATION"=w140:T3)  [unwired: 9 in]
        "Left Rear M" <- w140
        n65 = call <vilib>:"Translation_Create.vi"("Y"=w143, "X"=w145) -> ("TRANSLATION"=w139:T3)  [unwired: 9 in]
        "Right Rear M" <- w139
        n66 = call "Create_Trajectory_Value_Units_To_Meters.vi"("Units Selector"="Units Selector", "Units"=w134) -> ("Meters"=w133:dbl)  [unwired: 9 in]
        n67 = call <vilib>:"Translation_Create.vi"("Y"=w153, "X"=w155) -> ("TRANSLATION"=w141:T3)  [unwired: 9 in]
        "Right Front M" <- w141
        n68 = call <vilib>:"Translation_Create.vi"("Y"=w158, "X"=w161) -> ("TRANSLATION"=w160:T3)  [unwired: 9 in]
        "Left Front M" <- w160
        n69 = feedback-in #7("Field Selector") -> ()
        n70 = feedback #7("ZZZ" ("Field Selector")) -> (w120:string)
        n71 = call "Create_Trajectory_Value_Units_To_Meters.vi"("Units Selector"="Units Selector", "Units"=w131) -> ("Meters"=w130:dbl)  [unwired: 9 in]
        n72 = for {
          tunnel: "WayPoints" -> [w198] mode=indexing
          tunnel: [w197] -> w124 mode=indexing
          tunnel: "Units Selector" -> [w196]
          # "degrees -> radians\nUNITS -> meters\n\nweight unchanged"
          n73 = in-place {
            in-place-border: w196 -> [w199]
            n74 = in-place-cluster #8(w198) -> ("ANGLE"=w200:dbl, "X"=w205:dbl, "Y"=w203:dbl)
            n75 = call <vilib>:"Conv_Deg_Radians.vi"("Degress"=w200) -> ("Radians"=w201:dbl)  [unwired: 10 in]
            n76 = call "Create_Trajectory_Value_Units_To_Meters.vi"("Units Selector"=w199, "Units"=w205) -> ("Meters"=w204:dbl)  [unwired: 9 in]
            n77 = call "Create_Trajectory_Value_Units_To_Meters.vi"("Units Selector"=w199, "Units"=w203) -> ("Meters"=w202:dbl)  [unwired: 9 in]
            n78 = in-place-cluster #8("ANGLE"=w201, "X"=w204, "Y"=w202) -> (w197:T5)
          }
        }
        n79 = Reciprocal(x=w133) -> (1/x=w132:dbl)
        n80 = Reciprocal(x=w130) -> (1/x=w129:dbl)
        n81 = Not Equal?(x="Field Selector", y=w120) -> (x != y?=w116:bool)
        n82 = call "Create_Trajectory_Value_Units_To_Meters.vi"("Units Selector"="Units Selector", "Units"="MaxVelocity") -> ("Meters"=w164:dbl)  [unwired: 9 in]
        "MaxVelocity M/S" <- w164
        n83 = call "Create_Trajectory_Value_Units_To_Meters.vi"("Units Selector"="Units Selector", "Units"="MaxAcceleration") -> ("Meters"=w165:dbl)  [unwired: 9 in]
        "MaxAcceleration M/S^2" <- w165
        n84 = call "Create_Trajectory_Value_Units_To_Meters.vi"("Units Selector"="Units Selector", "Units"="Wheelbase Width") -> ("Meters"=w168:dbl)  [unwired: 9 in]
        "Wheelbase Width M" <- w168
        n85 = call "Create_Trajectory_Value_Units_To_Meters.vi"("Units Selector"="Units Selector", "Units"="Max Cent Accel") -> ("Meters"=w171:dbl)  [unwired: 9 in]
        "Max Cent Accel M/S^2" <- w171
        n86 = And(x=w114, y=w116) -> (x .and. y?=w115:bool)
        n87 = call <vilib>:"SimpleMotorFF_New.vi"("Ka"=w129, "Kv"=w132, "Ks"=w136) -> ("SIMPLE_MOTOR_FF"=w138:T4)  [unwired: 8 in]
        "SIMPLE_MOTOR_FF M" <- w138
        n88 = case shown="True" w115 {
          tunnel: "Field Selector" -> [_ w193]
          tunnel: w117 -> [_ w192]
          frame False {
          }
          frame True {
            n89 = call "Create_Trajectory_Get_Field_Info.vi"("Field Selector"=w193) -> ("File"=w194:string, "input cluster"=w191:T25)  [unwired: 9 in]
            n90 = call "Create_Trajectory_Read_Field_Pic.vi"("file name"=w194) -> ("Image Error"=w186:errorcluster, "Image Data"=w190:T6)  [unwired: 7 in, 2 out]
            n91 = case shown="Error .." w186 {
              frame Error {
                n92 = One Button Dialog(message="The field_picture file could not be read.  Execution will continue normally with a blank playing field.") -> ()  [unwired: 1 in, 1 out]
              }
              frame No Error {
              }
            }
            n93 = call "Create_Trajectory_Field_Crop_and_Scale.vi"("Disp Y Size Pixel"=430, "Disp X Size Pixel"=860, "Field Image"=w190, "field Info"=w191, "Display Image"=w192) -> ("Disp Image Out"=→"Field Display":T6)  [unwired: 5 in, 1 out]
          }
        }
        n94 = Wait (ms)(milliseconds to wait=u32 50) -> ()  [unwired: 1 out]
      }
      frame 1 {
        # "Read\nFile"
        # "Read config from trajectory File"
        n95 = call-poly <vilib>:"Read From XML File.vi"("XML File Path"="Read Config File Name") -> ("error out"=w224:errorcluster, "XML Elements"=w237:string)  [unwired: 8 in, 1 out]
        n96 = case shown="No Error" w224 {
          tunnel: w237 -> [w263 _]
          tunnel: w236 -> [w283 w406]
          tunnel: w235 -> [w282 w405]
          tunnel: w234 -> [w281 w404]
          tunnel: w233 -> [w280 w403]
          tunnel: w232 -> [w279 w402]
          tunnel: w231 -> [w278 w401]
          tunnel: [w277 w406] -> w230
          tunnel: [w276 w405] -> w229
          tunnel: [w275 w404] -> w228
          tunnel: [w274 w403] -> w227
          tunnel: [w273 w402] -> w226
          tunnel: [w272 w401] -> w225
          tunnel: w224 -> [w262 w400]
          tunnel: [w270 w400] -> w223
          tunnel: [w269 FALSE] -> w222
          tunnel: [w271 "" ("Write Config File Comment")] -> w221
          tunnel: [w268 w397] -> w220
          tunnel: w219 -> [w267 w397]
          tunnel: w218 -> [w264 w396]
          tunnel: [w266 w396] -> w217
          tunnel: [w260 w395] -> w216
          tunnel: w215 -> [w259 w395]
          tunnel: [w258 w394] -> w214
          tunnel: w213 -> [w257 w394]
          frame No Error {
            # "parse\nXML"
            # "A little bit of a \nkludge to read \nboth v2 and v1\nfile formats...."
            n97 = call "Create_Trajectory_Config_Parse_V1_V2_V3.vi"("error in (no error)"=w262, "Units Selector"=w264, "XML Elements"=w263) -> ("error out"=w265:errorcluster, "TrajCreateConfig"=w261:T14)  [unwired: 7 in]
            n98 = case shown="No Error" w265 {
              tunnel: w283 -> [_ w393]
              tunnel: w282 -> [_ w392]
              tunnel: w281 -> [_ w391]
              tunnel: w280 -> [_ w390]
              tunnel: w279 -> [_ w389]
              tunnel: w278 -> [_ w388]
              tunnel: [w354 w393] -> w277
              tunnel: [T13 {"TotalTImeSecs"=0.0, "States"=[]} ("TRAJECTORY") w392] -> w276
              tunnel: [w353 w391] -> w275
              tunnel: [w355 w390] -> w274
              tunnel: [FALSE w389] -> w273
              tunnel: [FALSE ("File Saved\nWithout\nError") w388] -> w272
              tunnel: w261 -> [w360 _]
              tunnel: [w332 "" ("Write Config File Comment")] -> w271
              tunnel: w265 -> [w358 w386]
              tunnel: [w358 w386] -> w270
              tunnel: [TRUE FALSE] -> w269
              tunnel: [FALSE ("File Saved\nWithout\nError") w384] -> w268
              tunnel: w267 -> [_ w384]
              tunnel: w264 -> [_ w383]
              tunnel: [w291 w383] -> w266
              tunnel: [w288 w382] -> w260
              tunnel: w259 -> [_ w382]
              tunnel: [FALSE ("File Saved\nWithout\nError") w381] -> w258
              tunnel: w257 -> [_ w381]
              frame No Error {
                # "This really doesn't do much\nstate 1 will write over this from\nthe user inputs....."
                # "Write to local\nuser controls"
                # "not used"
                # "not used"
                # "should make this a subvi"
                n99 = Unbundle By Name(w360) -> ("Write Config File Name"=w285:path, "Write Config File Comment"=w332:string, "WayPoints"=w354:T5[], "TRAJECTORY_CONFIG"=w353:T15, "IsCubic"=w355:bool, "Units Selector"=w291:T2, "UseWeights"=w288:bool)
                n100 = Unbundle By Name(w353) -> ("MaxVelocity"=w350:dbl, "Max Acceleration"=w349:dbl, "Reversed"=w348:bool, "DiffDrKineConstntDefined"=w347:bool, "CentAcellConstntDefined"=w346:bool, "DiffDrVoltConstntDefined"=w345:bool, "SwerveDrKineConstntDefined"=w344:bool, "MecanumDrKineConstntDefined"=w343:bool, "DIFF_DRIVE_KINE_CONSTRAINT"=w342:T16, "CENTRIPETAL_ACCEL_CONSTRAINT"=w339:T18, "DIFF_DRIVE_VOLTAGE_CONSTRAINT"=w336:T22, "MECANUM_DRIVE_KINE_CONSTRAINT"=w334:T23, "SWERVE_DRIVE_KINE_CONSTRAINT"=w333:T19)  [unwired: 2 out]
                n101 = Unbundle By Name(w334) -> ("MECA_DRIVE_KINEMATICS.FrontLeft"=w307:T3, "MECA_DRIVE_KINEMATICS.FrontRight"=w308:T3, "MECA_DRIVE_KINEMATICS.RearLeft"=w309:T3, "MECA_DRIVE_KINEMATICS.RearRight"=w310:T3)
                n102 = Unbundle By Name(w342) -> ("DIFF_DRIVE_KINEMATICS.TrackWidth_Meters"=w340:dbl)
                n103 = Unbundle By Name(w339) -> ("Max Cent Accel"=w337:dbl)
                n104 = Unbundle By Name(w336) -> ("Max Voltage"=w335:dbl, "SIMPLE_MOTOR_FF"=w293:T4)
                n105 = Unbundle By Name(w333) -> ("SwerveKinematics.Modules"=w327:T3[])
                n106 = Unbundle By Name(w293) -> ("Ks"=w302:dbl, "Kv"=w301:dbl, "Ka"=w294:dbl)
                n107 = for {
                  tunnel: w354 -> [w371] mode=indexing
                  tunnel: [w370] -> w290 mode=indexing
                  tunnel: w291 -> [w369]
                  # "radians -> degrees\nmeters -> inches\nWeights stay the same"
                  n108 = in-place {
                    in-place-border: w369 -> [w372]
                    n109 = in-place-cluster #9(w371) -> ("ANGLE"=w373:dbl, "X"=w378:dbl, "Y"=w376:dbl)
                    n110 = call "Create_Trajectory_Value_Meters_To_Units.vi"("Units Selector"=w372, "Meters"=w376) -> ("Units"=w375:dbl)  [unwired: 9 in]
                    n111 = call <vilib>:"Conv_Radians_Deg.vi"("Radians"=w373) -> ("Degrees"=w374:dbl)  [unwired: 10 in]
                    n112 = call "Create_Trajectory_Value_Meters_To_Units.vi"("Units Selector"=w372, "Meters"=w378) -> ("Units"=w377:dbl)  [unwired: 9 in]
                    n113 = in-place-cluster #9("ANGLE"=w374, "X"=w377, "Y"=w375) -> (w370:T5)
                  }
                }
                n114 = case shown="True" w355 {
                  tunnel: [enum32{"Radio Selection 1", "Radio Selection 2"}."Radio Selection 2" ("Spline Type") enum32{"Radio Selection 1", "Radio Selection 2"}."Radio Selection 1" ("Spline Type")] -> w356
                  frame False {
                  }
                  frame True {
                  }
                }
                n115 = Reciprocal(x=w301) -> (1/x=w300:dbl)
                n116 = Reciprocal(x=w294) -> (1/x=w297:dbl)
                n117 = call "ChangeFileExtension.vi"("NewExtenion"=".json", "In FileName"=w285) -> ("Out FileName"=w284:path)  [unwired: 9 in]
                n118 = call "ChangeFileExtension.vi"("NewExtenion"=".csv", "In FileName"=w285) -> ("Out FileName"=w331:path)  [unwired: 9 in]
                n119 = call <vilib>:"Translation_GetXY.vi"("In Translation"=w307) -> ("Y"=w324:dbl, "X"=w326:dbl)  [unwired: 9 in]
                n120 = call <vilib>:"Translation_GetXY.vi"("In Translation"=w308) -> ("Y"=w320:dbl, "X"=w322:dbl)  [unwired: 9 in]
                n121 = call <vilib>:"Translation_GetXY.vi"("In Translation"=w309) -> ("Y"=w316:dbl, "X"=w318:dbl)  [unwired: 9 in]
                n122 = for {
                  tunnel: w327 -> [w364] mode=indexing
                  tunnel: [w363] -> w328 mode=indexing
                  tunnel: w291 -> [w362]
                  n123 = call <vilib>:"Translation_GetXY.vi"("In Translation"=w364) -> ("Y"=w366:dbl, "X"=w368:dbl)  [unwired: 9 in]
                  n124 = call "Create_Trajectory_Value_Meters_To_Units.vi"("Units Selector"=w362, "Meters"=w368) -> ("Units"=w367:dbl)  [unwired: 9 in]
                  n125 = call "Create_Trajectory_Value_Meters_To_Units.vi"("Units Selector"=w362, "Meters"=w366) -> ("Units"=w365:dbl)  [unwired: 9 in]
                  n126 = call <vilib>:"Translation_Create.vi"("Y"=w365, "X"=w367) -> ("TRANSLATION"=w363:T3)  [unwired: 9 in]
                }
                n127 = call <vilib>:"Translation_GetXY.vi"("In Translation"=w310) -> ("Y"=w312:dbl, "X"=w314:dbl)  [unwired: 9 in]
                n128 = call "Create_Trajectory_Value_Meters_To_Units.vi"("Units Selector"=w291, "Meters"=w300) -> ("Units"=w299:dbl)  [unwired: 9 in]
                n129 = call "Create_Trajectory_Value_Meters_To_Units.vi"("Units Selector"=w291, "Meters"=w350) -> ("Units"=w351:dbl)  [unwired: 9 in]
                n130 = call "Create_Trajectory_Value_Meters_To_Units.vi"("Units Selector"=w291, "Meters"=w297) -> ("Units"=w296:dbl)  [unwired: 9 in]
                n131 = local write "Trajectory JSON File Name"(w284) -> ()
                n132 = local write "Trajectory CSV File Name"(w331) -> ()
                n133 = call "Create_Trajectory_Value_Meters_To_Units.vi"("Units Selector"=w291, "Meters"=w326) -> ("Units"=w325:dbl)  [unwired: 9 in]
                n134 = call "Create_Trajectory_Value_Meters_To_Units.vi"("Units Selector"=w291, "Meters"=w349) -> ("Units"=w352:dbl)  [unwired: 9 in]
                n135 = call "Create_Trajectory_Value_Meters_To_Units.vi"("Units Selector"=w291, "Meters"=w322) -> ("Units"=w321:dbl)  [unwired: 9 in]
                n136 = local write "Units Selector"(w291) -> ()
                n137 = local write "UseWeights"(w288) -> ()
                n138 = local write "Write Config File Name"(w285) -> ()
                n139 = local write "Write Config File Comment"(w332) -> ()
                n140 = local write "Trajectory File Comment"(w332) -> ()
                n141 = call "Create_Trajectory_Value_Meters_To_Units.vi"("Units Selector"=w291, "Meters"=w318) -> ("Units"=w317:dbl)  [unwired: 9 in]
                n142 = Reciprocal(x=w299) -> (1/x=w298:dbl)
                n143 = call "Create_Trajectory_Value_Meters_To_Units.vi"("Units Selector"=w291, "Meters"=w314) -> ("Units"=w313:dbl)  [unwired: 9 in]
                n144 = Reciprocal(x=w296) -> (1/x=w295:dbl)
                n145 = call "Create_Trajectory_Value_Meters_To_Units.vi"("Units Selector"=w291, "Meters"=w324) -> ("Units"=w323:dbl)  [unwired: 9 in]
                n146 = call "Create_Trajectory_Value_Meters_To_Units.vi"("Units Selector"=w291, "Meters"=w320) -> ("Units"=w319:dbl)  [unwired: 9 in]
                n147 = local write "Use Mecanum \nDrive Kinematics\nConstraint"(w343) -> ()
                n148 = call "Create_Trajectory_Value_Meters_To_Units.vi"("Units Selector"=w291, "Meters"=w316) -> ("Units"=w315:dbl)  [unwired: 9 in]
                n149 = call "Create_Trajectory_Value_Meters_To_Units.vi"("Units Selector"=w291, "Meters"=w312) -> ("Units"=w311:dbl)  [unwired: 9 in]
                n150 = call "Create_Trajectory_Value_Meters_To_Units.vi"("Units Selector"=w291, "Meters"=w340) -> ("Units"=w341:dbl)  [unwired: 9 in]
                n151 = call "Create_Trajectory_Value_Meters_To_Units.vi"("Units Selector"=w291, "Meters"=w337) -> ("Units"=w338:dbl)  [unwired: 9 in]
                n152 = local write "Use Swerve Drive\nKinematics\nConstraint"(w344) -> ()
                n153 = local write "Use Centripetal\nAcceleration\nConstaint"(w346) -> ()
                n154 = call <vilib>:"SimpleMotorFF_New.vi"("Ka"=w295, "Kv"=w298, "Ks"=w302) -> ("SIMPLE_MOTOR_FF"=w292:T4)  [unwired: 8 in]
                n155 = local write "Use Diff Drive\nKinematic\nConstraint"(w347) -> ()
                n156 = local write "MaxVelocity"(w351) -> ()
                n157 = local write "MaxAcceleration"(w352) -> ()
                n158 = local write "Spline Type"(w356) -> ()
                n159 = call <vilib>:"Translation_Create.vi"("Y"=w323, "X"=w325) -> ("TRANSLATION"=w306:T3)  [unwired: 9 in]
                n160 = local write "Use Diff Drive\nVoltage\nConstraint"(w345) -> ()
                n161 = call <vilib>:"Translation_Create.vi"("Y"=w319, "X"=w321) -> ("TRANSLATION"=w305:T3)  [unwired: 9 in]
                n162 = call <vilib>:"Translation_Create.vi"("Y"=w315, "X"=w317) -> ("TRANSLATION"=w304:T3)  [unwired: 9 in]
                n163 = call <vilib>:"Translation_Create.vi"("Y"=w311, "X"=w313) -> ("TRANSLATION"=w303:T3)  [unwired: 9 in]
                n164 = local write "Reverse"(w348) -> ()
                n165 = local write "Wheelbase Width"(w341) -> ()
                n166 = local write "Max Cent Accel"(w338) -> ()
                n167 = local write "SIMPLE_MOTOR_FF"(w292) -> ()
                n168 = local write "Max Voltage"(w335) -> ()
                n169 = local write "WayPoints"(w290) -> ()
                n170 = local write "Left Front"(w306) -> ()
                n171 = local write "Right Front"(w305) -> ()
                n172 = local write "Right Rear"(w303) -> ()
                n173 = local write "Left Rear"(w304) -> ()
                n174 = local write "Wheels"(w328) -> ()
              }
              frame Error {
              }
            }
          }
          frame Error {
          }
        }
        "Config File Read\nWithout Error" <- w222
        "Config File  Read Error" <- w223
        "Read Config File Comment" <- w221
      }
      frame 2 {
        w407 = FALSE ("File Saved\nWithout\nError")
        # "#TODO  If differential speed is exceeded, flag an error."
        # "Waypoints"
        # "diff max speed\nexceeded."
        # "Inches/Sec"
        # "Inches"
        # "Input was Inches, plot inches...."
        # "max velocity"
        # "Create Trajectory"
        # "allow a little excess"
        # "in meters"
        # "Diff drive"
        # "Distance\nVelocity\nAcceleration\nRotatonal Velocity\nHeading\nJerk (Delta Accel)"
        # "FIELD POSITION\nGRAPH"
        # "GRAPH OF DATA"
        # "construct the trajectory\nconfiguration information"
        # "trajectory \nmeters, radians"
        # "DIFFERENTIAL DRIVE MAX SPEED"
        # "Create absolute Trajectory\nStates"
        n175 = call <vilib>:"TrajectoryConfig_Create.vi"("MaxAcceleration"=w423, "MaxVelocity"=w422) -> ("TRAJECTORY_CONFIG"=w439:T15)  [unwired: 9 in]
        n176 = call <vilib>:"TrajectoryConfig_setReversed.vi"("Reversed"=w424, "inTRAJECTORY_CONFIG"=w439) -> ("outTRAJECTORY_CONFIG"=w438:T15)  [unwired: 9 in]
        n177 = call <vilib>:"DiffKinematics_New.vi"("TrackWidth_Meters"=w425) -> ("DIFF_DRIVE_KINEMATICS"=w452:T17)  [unwired: 10 in]
        n178 = case shown="True" w416 {
          tunnel: w438 -> [w583 w586]
          tunnel: [w583 w585] -> w480
          tunnel: w452 -> [_ w584]
          frame False {
          }
          frame True {
            n179 = call <vilib>:"TrajectoryConfig_setKinematicsDiffDrive.vi"("DIFF_DRIVE_KINEMATICS"=w584, "inTRAJECTORY_CONFIG"=w586) -> ("outTRAJECTORY_CONFIG"=w585:T15)  [unwired: 9 in]
          }
        }
        n180 = for {
          tunnel: w413 -> [w494] mode=indexing
          tunnel: [w491] -> w412 mode=indexing
          tunnel: [w490] -> w411 mode=indexing
          n181 = Unbundle By Name(w494) -> ("X"=w493:dbl, "Y"=w492:dbl)
          n182 = call <vilib>:"Conv_Meters_Inches.vi"("Meters"=w493) -> ("Inches"=w491:dbl)  [unwired: 10 in]
          n183 = call <vilib>:"Conv_Meters_Inches.vi"("Meters"=w492) -> ("Inches"=w490:dbl)  [unwired: 10 in]
        }
        n184 = case shown="True" w426 {
          tunnel: w480 -> [w579 w582]
          tunnel: w427 -> [_ w581]
          tunnel: [w579 w580] -> w460
          frame False {
          }
          frame True {
            n185 = call <vilib>:"TrajectoryConfig_setCentripetalAccel.vi"("Max Cent Accel"=w581, "inTRAJECTORY_CONFIG"=w582) -> ("outTRAJECTORY_CONFIG"=w580:T15)  [unwired: 9 in]
          }
        }
        n186 = case shown="True" w428 {
          tunnel: w460 -> [w537 w543]
          tunnel: [w537 w542] -> w459
          tunnel: w429 -> [_ w541]
          tunnel: w425 -> [_ w540]
          tunnel: w430 -> [_ w538]
          frame False {
          }
          frame True {
            n187 = call <vilib>:"DiffKinematics_New.vi"("TrackWidth_Meters"=w540) -> ("DIFF_DRIVE_KINEMATICS"=w539:T17)  [unwired: 10 in]
            n188 = call <vilib>:"TrajectoryConfig_setVoltageDiffDrive.vi"("SIMPLE_MOTOR_FF"=w541, "DIFF_DRIVE_KINEMATICS"=w539, "Max Voltage"=w538, "inTRAJECTORY_CONFIG"=w543) -> ("outTRAJECTORY_CONFIG"=w542:T15)  [unwired: 7 in]
          }
        }
        n189 = case shown="True" w431 {
          tunnel: [w532 w536] -> w448
          tunnel: w459 -> [w532 w535]
          tunnel: w432 -> [_ w533]
          frame False {
          }
          frame True {
            n190 = call <vilib>:"SwerveKinematics_NewX.vi"("Wheels"=w533) -> ("SWERVE_DRIVE_KINEMATICS"=w534:T20)  [unwired: 10 in]
            n191 = call <vilib>:"TrajectoryConfig_setKinematicsSwerveDrive.vi"("SWERVE_DRIVE_KINEMATICS"=w534, "inTRAJECTORY_CONFIG"=w535) -> ("outTRAJECTORY_CONFIG"=w536:T15)  [unwired: 9 in]
          }
        }
        n192 = case shown="True" w436 {
          tunnel: [w495 w502] -> w421
          tunnel: w448 -> [w495 w501]
          tunnel: w435 -> [_ w499]
          tunnel: w434 -> [_ w498]
          tunnel: w433 -> [_ w497]
          tunnel: w437 -> [_ w496]
          frame False {
          }
          frame True {
            n193 = call <vilib>:"MecaKinematics_New.vi"("RearRight"=w496, "RearLeft"=w497, "FrontRight"=w498, "FrontLeft"=w499) -> ("MECA_DRIVE_KINEMATICS"=w500:T24)  [unwired: 7 in]
            n194 = call <vilib>:"TrajectoryConfig_setKinematicsMecanumDrive.vi"("MECA_DRIVE_KINEMATICS"=w500, "inTRAJECTORY_CONFIG"=w501) -> ("outTRAJECTORY_CONFIG"=w502:T15)  [unwired: 9 in]
          }
        }
        n195 = case shown="\"Radio Selection 1\", Default" "Spline Type" {
          tunnel: [w555 w564] -> w445
          tunnel: w421 -> [w554 w561]
          tunnel: [w556 w563] -> w420
          tunnel: [TRUE FALSE] -> w419
          tunnel: w413 -> [w552 w559]
          tunnel: w408 -> [w546 w557]
          frame "Radio Selection 1", Default {
            # "format\nwaypoints for\nspline functions"
            # "Calc\ncubic\nsplines"
            n196 = call <vilib>:"Util_WeightedWaypoint_To_WeightedWayPoint.vi"("DisplayWeightedWayPoints"=w552) -> ("WeightedWayPoints"=w551:T26[])  [unwired: 10 in]
            n197 = call <vilib>:"SplineHelp_GetCubicCtrlVectorsFromWeightedWayPts.vi"("Use Weights"=w546, "WeightedWayPoints"=w551) -> ("Interior WAYPOINTS"=w550:T3[], "SplineControlVectors"=w549:T27[])  [unwired: 8 in]
            n198 = Index Array(array=w549, index #1=0 ("index"), index #2=1 ("index")) -> (element #1=w548:T27, element #2=w547:T27)
            n199 = call <vilib>:"TrajectoryGenerate_Make_Cubic_CtrlVect.vi"("traj_config"=w554, "end-Spline_Ctrl_Vector"=w547, "Interior WAYPOINTS"=w550, "initial-Spline_Ctrl_Vector"=w548) -> ("error out"=w555:errorcluster, "TRAJECTORY"=w556:T13)  [unwired: 6 in]
          }
          frame "Radio Selection 2" {
            # "format\nwaypoints for\nspline functions"
            # "CALC\nQUINTIC\nSPLINE"
            n200 = call <vilib>:"Util_WeightedWaypoint_To_WeightedWayPoint.vi"("DisplayWeightedWayPoints"=w559) -> ("WeightedWayPoints"=w558:T26[])  [unwired: 10 in]
            n201 = call <vilib>:"SplineHelp_GetQuinticCtrlVectorsFromWeightedWayPts.vi"("Use Weights"=w557, "WayPoints"=w558) -> ("SplineControlVectors"=w560:T27[])  [unwired: 9 in]
            n202 = call <vilib>:"TrajectoryGenerate_Make_Quintic_CtrlVect.vi"("traj_config"=w561, "input_ControlVectors"=w560) -> ("error out"=w564:errorcluster, "TRAJECTORY"=w563:T13)  [unwired: 8 in]
          }
        }
        "Trajectory calculation error" <- w445
        n203 = Unbundle By Name(w420) -> ("States"=w451:T7[], "TotalTImeSecs"=w455:dbl)
        "Trajectory States" <- w451
        n204 = while {
          tunnel: [w524] -> w457 mode=indexing
          tunnel: [w515] -> w476 mode=indexing
          tunnel: [w517] -> w475 mode=indexing
          tunnel: [w521] -> w474 mode=indexing
          tunnel: [w516] -> w473 mode=indexing
          tunnel: [w531] -> w472 mode=indexing
          shift-right: [w525] -> _
          shift-left: 0.0 -> [w515]
          tunnel: [w519] -> w456 mode=indexing
          tunnel: w455 -> [w511]
          tunnel: w420 -> [w503]
          i -> [w509]
          stop <- w510 stop-if-true
          # "Time Df"
          # "Jerk"
          # "Dist"
          n205 = To Double Precision Float(number=w509) -> (double precision float=w508:dbl)
          n206 = Multiply(x=w508, y=0.02) -> (x*y=w506:dbl)
          n207 = feedback #10(0.0 ("TimeSeconds")) -> (w527:dbl)
          n208 = feedback #11(0.0 ("TimeSeconds")) -> (w529:dbl)
          n209 = feedback #12(0.0 ("TimeSeconds")) -> (w522:dbl)
          n210 = call <vilib>:"Trajectory_Sample.vi"("Time"=w506, "InputTRAJECTORY"=w503) -> ("OutputTRAJ_STATE"=w504:T7)  [unwired: 9 in]
          n211 = call <vilib>:"Util_TrajectoryState_Meters_To_Inches.vi"("absTRAJECTORY"=w504) -> ("outputRelativeTRAJECTORY"=w505:T7)  [unwired: 10 in]
          n212 = Unbundle By Name(w505) -> ("TimeSeconds"=w524:dbl, "Velocity"=w517:dbl, "Acceleration"=w521:dbl, "Curvature"=w518:dbl, "POSE.ROTATION.VALUE"=w531:dbl)
          n213 = feedback-in #10(w517) -> ()
          n214 = feedback-in #11(w524) -> ()
          n215 = feedback-in #12(w521) -> ()
          n216 = Add(x=w517, y=w527) -> (x+y=w526:dbl)
          n217 = Subtract(x=w524, y=w529) -> (x-y=w512:dbl)
          n218 = Subtract(x=w521, y=w522) -> (x-y=w520:dbl)
          n219 = Compound Arithmetic op=MULTIPLY(w526, 0.5 ("value"), w512) -> (w514:dbl)
          n220 = Divide(x=w520, y=w512) -> (x/y=w519:dbl)
          n221 = Add(x=w514, y=w515) -> (x+y=w525:dbl)
          n222 = Greater Or Equal?(x=w506, y=w511) -> (x >= y?=w510:bool)
          n223 = Multiply(x=w517, y=w518) -> (x*y=w516:dbl)
        }
        n224 = for {
          tunnel: w451 -> [w569] mode=indexing
          tunnel: w425 -> [w578]
          tunnel: [w576] -> w467 mode=indexing
          tunnel: [w575] -> w466 mode=indexing
          tunnel: [w572] -> w465 mode=indexing
          tunnel: [w570] -> w464 mode=indexing
          tunnel: [w566] -> w454 mode=indexing
          tunnel: [w565] -> w453 mode=indexing
          n225 = Unbundle By Name(w569) -> ("POSE.TRANSLATION.X"=w568:dbl, "POSE.TRANSLATION.Y"=w567:dbl)
          n226 = call <vilib>:"Util_TrajState_to_DiffDrive_WheelPos.vi"("Wheelbase"=w578, "TRAJ_STATE"=w569) -> ("Right Y"=w571:dbl, "Right X"=w573:dbl, "Left Y"=w574:dbl, "Left X"=w577:dbl)  [unwired: 6 in]
          n227 = call <vilib>:"Conv_Meters_Inches.vi"("Meters"=w577) -> ("Inches"=w576:dbl)  [unwired: 10 in]
          n228 = call <vilib>:"Conv_Meters_Inches.vi"("Meters"=w573) -> ("Inches"=w572:dbl)  [unwired: 10 in]
          n229 = call <vilib>:"Conv_Meters_Inches.vi"("Meters"=w568) -> ("Inches"=w565:dbl)  [unwired: 10 in]
          n230 = call <vilib>:"Conv_Meters_Inches.vi"("Meters"=w574) -> ("Inches"=w575:dbl)  [unwired: 10 in]
          n231 = call <vilib>:"Conv_Meters_Inches.vi"("Meters"=w571) -> ("Inches"=w570:dbl)  [unwired: 10 in]
          n232 = call <vilib>:"Conv_Meters_Inches.vi"("Meters"=w567) -> ("Inches"=w566:dbl)  [unwired: 10 in]
        }
        n233 = for {
          tunnel: [w588] -> w487 mode=indexing
          tunnel: [w587] -> w485 mode=indexing
          tunnel: w451 -> [w595] mode=indexing
          tunnel: w452 -> [w589]
          # "see if max speed violated  by\neither wheel speed"
          n234 = Unbundle By Name(w595) -> ("Velocity"=w593:dbl, "Curvature"=w594:dbl)
          n235 = Multiply(x=w593, y=w594) -> (x*y=w591:dbl)
          n236 = call <vilib>:"ChassisSpeeds_New.vi"("vAngular"=w591, "vY"=0.0, "vX"=w593) -> ("CHASSIS"=w590:T28)  [unwired: 8 in]
          n237 = call <vilib>:"DiffKinematics_toWheelSpeed.vi"("CHASSIS Speed"=w590, "DIFF_DRIVE_KINEMATICS"=w589) -> ("RightVelocity"=w587:dbl, "LeftVelocity"=w588:dbl)  [unwired: 8 in]
        }
        n238 = Bundle(w412, w411) -> (w410:cluster{dbl[], dbl[]})  [unwired: 1 in]
        n239 = Bundle(w453, w454) -> (w462:cluster{dbl[], dbl[]})  [unwired: 1 in]
        n240 = Bundle(w467, w466) -> (w461:cluster{dbl[], dbl[]})  [unwired: 1 in]
        n241 = Bundle(w465, w464) -> (w463:cluster{dbl[], dbl[]})  [unwired: 1 in]
        n242 = Absolute Value(x=w487) -> (abs(x)=w486:dbl[])
        n243 = Absolute Value(x=w485) -> (abs(x)=w484:dbl[])
        n244 = Multiply(x=w422, y=1.01) -> (x*y=w446:dbl)
        n245 = Build Array(w462, w461, w463, w410) -> (→"Position":cluster{dbl[], dbl[]}[])
        n246 = Array Max & Min(array=w486) -> (max value=w482:dbl)  [unwired: 3 out]
        n247 = Array Max & Min(array=w484) -> (max value=w481:dbl)  [unwired: 3 out]
        n248 = Greater?(x=w482, y=w446) -> (0:w488:bool)
        n249 = Greater?(x=w481, y=w446) -> (0:w483:bool)
        n250 = Max & Min(x=w482, y=w481) -> (max(x,y)=w450:dbl)  [unwired: 1 out]
        n251 = Bundle(w457, w473) -> (w471:cluster{dbl[], dbl[]})  [unwired: 1 in]
        n252 = Bundle(w457, w472) -> (w470:cluster{dbl[], dbl[]})  [unwired: 1 in]
        n253 = Bundle(w457, w475) -> (w478:cluster{dbl[], dbl[]})  [unwired: 1 in]
        n254 = Bundle(w457, w456) -> (w458:cluster{dbl[], dbl[]})  [unwired: 1 in]
        n255 = Bundle(w457, w476) -> (w479:cluster{dbl[], dbl[]})  [unwired: 1 in]
        n256 = Bundle(w457, w474) -> (w477:cluster{dbl[], dbl[]})  [unwired: 1 in]
        n257 = Compound Arithmetic op=OR(w488, w483) -> (w417:bool)
        n258 = call <vilib>:"Conv_Meters_Inches.vi"("Meters"=w450) -> ("Inches"=→"differential \ndrive \nmax speed":dbl)  [unwired: 10 in]
        n259 = Array Size(array=w451) -> (size(s)=w443:i32)
        "Traj States\nSize" <- w443
        n260 = Build Array(w479, w478, w477, w471, w470, w458) -> (→"Trajectory Data":cluster{dbl[], dbl[]}[])
        n261 = And(x=w417, y=w416) -> (x .and. y?=w415:bool)
        n262 = Not(x=w415) -> (.not. x?=w441:bool)
        n263 = Greater Than 0?(x=w443) -> (x > 0?=w442:bool)
        n264 = And(x=w442, y=w441) -> (x .and. y?=w444:bool)
      }
      frame 3 {
        # "Write trajectory to CSV File"
        n265 = case shown="\"Radio Selection 1\", Default" w596 {
          tunnel: w624 -> [w634 w636]
          tunnel: [w633 w636] -> w628
          tunnel: [TRUE FALSE] -> w626
          frame "Radio Selection 1", Default {
            # "Relative"
            n266 = call <vilib>:"Util_Trajectory_Absolute_To_Relative.vi"("absTRAJECTORY"=w634) -> ("outputRelativeTRAJECTORY"=w633:T13)  [unwired: 10 in]
          }
          frame "Radio Selection 2" {
            # "Absolute"
          }
        }
        n267 = call <vilib>:"Util_Trajectory_WriteFile.vi"("Trajectory is Cubic"=w622, "UseWeights"=w598, "Trajectory Is Relative"=w626, "TRAJECTORY_CONFIG"=w623, "UtilityWayPoints"=w599, "TRAJECTORY"=w628, "Comment"="Trajectory File Comment", "Trajectory File Name"="Trajectory CSV File Name") -> ("error out"=w627:errorcluster)  [unwired: 3 in]
        "Write Trajectory\nFile Error" <- w627
        n268 = local write "Write Config File Comment"("Trajectory File Comment") -> ()
        n269 = case shown="Error .." w627 {
          tunnel: [TRUE ("File Saved\nWithout\nError") FALSE ("File Saved\nWithout\nError")] -> w620
          frame No Error {
          }
          frame Error {
          }
        }
      }
      frame 4 {
        # "Write trajectory to JSON File"
        n270 = case shown="\"Radio Selection 1\", Default" w645 {
          tunnel: w672 -> [w772 w774]
          tunnel: [w771 w774] -> w641
          tunnel: [TRUE FALSE] -> _
          frame "Radio Selection 1", Default {
            # "Relative"
            n271 = call <vilib>:"Util_Trajectory_Absolute_To_Relative.vi"("absTRAJECTORY"=w772) -> ("outputRelativeTRAJECTORY"=w771:T13)  [unwired: 10 in]
          }
          frame "Radio Selection 2" {
            # "Absolute"
          }
        }
        n272 = Unbundle By Name(w641) -> ("States"=w640:T7[])
        n273 = case shown="\"Radio Selection 1\"" "PathWeaver Length Units" {
          tunnel: w640 -> [w674 w675 w699 w729 w749]
          tunnel: [w674 w676 w698 w728 w748] -> w637
          frame "Radio Selection 1" {
            # "Meters - do nothing"
          }
          frame "Radio Selection 2" {
            # "Conv Meters to Centimeters"
            n274 = for {
              tunnel: w675 -> [w678] mode=indexing
              tunnel: [w677] -> w676 mode=indexing
              n275 = in-place {
                n276 = in-place-cluster #13(w678) -> ("Acceleration"=w689:dbl, "TimeSeconds"=w697:dbl, "Velocity"=w687:dbl, "Curvature"=w692:dbl, "POSE.TRANSLATION.X"=w679:dbl, "POSE.TRANSLATION.Y"=w683:dbl, "POSE.ROTATION.VALUE"=w694:dbl, "POSE.ROTATION.COS"=w696:dbl, "POSE.ROTATION.SIN"=w695:dbl)
                n277 = Multiply(x=w679, y=100.0) -> (x*y=w680:dbl)
                n278 = Multiply(x=w683, y=100.0) -> (x*y=w682:dbl)
                n279 = Multiply(x=w687, y=100.0) -> (x*y=w686:dbl)
                n280 = Multiply(x=w689, y=100.0) -> (x*y=w690:dbl)
                n281 = Divide(x=w692, y=100.0 ("Centimeter")) -> (x/y=w693:dbl)
                n282 = in-place-cluster #13("Acceleration"=w690, "TimeSeconds"=w697, "Velocity"=w686, "Curvature"=w693, "POSE.TRANSLATION.X"=w680, "POSE.TRANSLATION.Y"=w682, "POSE.ROTATION.VALUE"=w694, "POSE.ROTATION.COS"=w696, "POSE.ROTATION.SIN"=w695) -> (w677:T7)
              }
            }
          }
          frame "Radio Selection 3" {
            # "Who uses yards ????"
            # "Conv Meters to Yards"
            n283 = for {
              tunnel: w699 -> [w701] mode=indexing
              tunnel: [w700] -> w698 mode=indexing
              n284 = in-place {
                n285 = in-place-cluster #14(w701) -> ("Acceleration"=w721:dbl, "TimeSeconds"=w727:dbl, "Velocity"=w722:dbl, "Curvature"=w719:dbl, "POSE.TRANSLATION.X"=w723:dbl, "POSE.TRANSLATION.Y"=w724:dbl, "POSE.ROTATION.VALUE"=w720:dbl, "POSE.ROTATION.COS"=w726:dbl, "POSE.ROTATION.SIN"=w725:dbl)
                n286 = call <vilib>:"Conv_Meters_Feet.vi"("Meters"=w724) -> ("Feet"=w706:dbl)  [unwired: 10 in]
                n287 = call <vilib>:"Conv_Meters_Feet.vi"("Meters"=w721) -> ("Feet"=w716:dbl)  [unwired: 10 in]
                n288 = call <vilib>:"Conv_Meters_Feet.vi"("Meters"=w722) -> ("Feet"=w712:dbl)  [unwired: 10 in]
                n289 = call <vilib>:"Conv_Meters_Feet.vi"("Meters"=w723) -> ("Feet"=w703:dbl)  [unwired: 10 in]
                n290 = Divide(x=w703, y=3.0) -> (x/y=w702:dbl)
                n291 = Divide(x=w706, y=3.0) -> (x/y=w705:dbl)
                n292 = Divide(x=w716, y=3.0) -> (x/y=w714:dbl)
                n293 = Divide(x=w712, y=3.0) -> (x/y=w711:dbl)
                n294 = call <vilib>:"Conv_Meters_Feet.vi"("Meters"=1.0 ("Centimeter")) -> ("Feet"=w708:dbl)  [unwired: 10 in]
                n295 = Divide(x=w708, y=3.0) -> (x/y=w709:dbl)
                n296 = Divide(x=w719, y=w709) -> (x/y=w718:dbl)
                n297 = in-place-cluster #14("Acceleration"=w714, "TimeSeconds"=w727, "Velocity"=w711, "Curvature"=w718, "POSE.TRANSLATION.X"=w702, "POSE.TRANSLATION.Y"=w705, "POSE.ROTATION.VALUE"=w720, "POSE.ROTATION.COS"=w726, "POSE.ROTATION.SIN"=w725) -> (w700:T7)
              }
            }
          }
          frame "Radio Selection 4" {
            # "Meters Conv to Feet"
            n298 = for {
              tunnel: w729 -> [w731] mode=indexing
              tunnel: [w730] -> w728 mode=indexing
              n299 = in-place {
                n300 = in-place-cluster #15(w731) -> ("Acceleration"=w739:dbl, "TimeSeconds"=w747:dbl, "Velocity"=w741:dbl, "Curvature"=w733:dbl, "POSE.TRANSLATION.X"=w743:dbl, "POSE.TRANSLATION.Y"=w744:dbl, "POSE.ROTATION.VALUE"=w736:dbl, "POSE.ROTATION.COS"=w746:dbl, "POSE.ROTATION.SIN"=w745:dbl)
                n301 = call <vilib>:"Conv_Meters_Feet.vi"("Meters"=w739) -> ("Feet"=w738:dbl)  [unwired: 10 in]
                n302 = call <vilib>:"Conv_Meters_Feet.vi"("Meters"=w741) -> ("Feet"=w740:dbl)  [unwired: 10 in]
                n303 = call <vilib>:"Conv_Meters_Feet.vi"("Meters"=w743) -> ("Feet"=w742:dbl)  [unwired: 10 in]
                n304 = call <vilib>:"Conv_Meters_Feet.vi"("Meters"=w744) -> ("Feet"=w737:dbl)  [unwired: 10 in]
                n305 = call <vilib>:"Conv_Meters_Feet.vi"("Meters"=1.0 ("Centimeter")) -> ("Feet"=w734:dbl)  [unwired: 10 in]
                n306 = Divide(x=w733, y=w734) -> (x/y=w732:dbl)
                n307 = in-place-cluster #15("Acceleration"=w738, "TimeSeconds"=w747, "Velocity"=w740, "Curvature"=w732, "POSE.TRANSLATION.X"=w742, "POSE.TRANSLATION.Y"=w737, "POSE.ROTATION.VALUE"=w736, "POSE.ROTATION.COS"=w746, "POSE.ROTATION.SIN"=w745) -> (w730:T7)
              }
            }
          }
          frame "Radio Selection 5" {
            # "Meters - Conv to Inches"
            n308 = for {
              tunnel: w749 -> [w751] mode=indexing
              tunnel: [w750] -> w748 mode=indexing
              n309 = in-place {
                n310 = in-place-cluster #16(w751) -> ("Acceleration"=w759:dbl, "TimeSeconds"=w767:dbl, "Velocity"=w761:dbl, "Curvature"=w753:dbl, "POSE.TRANSLATION.X"=w763:dbl, "POSE.TRANSLATION.Y"=w764:dbl, "POSE.ROTATION.VALUE"=w756:dbl, "POSE.ROTATION.COS"=w766:dbl, "POSE.ROTATION.SIN"=w765:dbl)
                n311 = call <vilib>:"Conv_Meters_Inches.vi"("Meters"=w759) -> ("Inches"=w758:dbl)  [unwired: 10 in]
                n312 = call <vilib>:"Conv_Meters_Inches.vi"("Meters"=w761) -> ("Inches"=w760:dbl)  [unwired: 10 in]
                n313 = call <vilib>:"Conv_Meters_Inches.vi"("Meters"=w763) -> ("Inches"=w762:dbl)  [unwired: 10 in]
                n314 = call <vilib>:"Conv_Meters_Inches.vi"("Meters"=w764) -> ("Inches"=w757:dbl)  [unwired: 10 in]
                n315 = call <vilib>:"Conv_Meters_Inches.vi"("Meters"=1.0 ("Centimeter")) -> ("Inches"=w754:dbl)  [unwired: 10 in]
                n316 = Divide(x=w753, y=w754) -> (x/y=w752:dbl)
                n317 = in-place-cluster #16("Acceleration"=w758, "TimeSeconds"=w767, "Velocity"=w760, "Curvature"=w752, "POSE.TRANSLATION.X"=w762, "POSE.TRANSLATION.Y"=w757, "POSE.ROTATION.VALUE"=w756, "POSE.ROTATION.COS"=w766, "POSE.ROTATION.SIN"=w765) -> (w750:T7)
              }
            }
          }
        }
        n318 = call <vilib>:"Trajectory_New.vi"("TRAJ_STATES"=w637) -> ("TRAJECTORY"=w638:T13)  [unwired: 10 in]
        n319 = Path To String(path="Trajectory JSON File Name") -> (string=w643:string)
        n320 = call <vilib>:"TrajectoryUtil_toPathWeaverJSON.vi"("inTRAJECTORY"=w638, "FileName"=w643) -> ("error out"=w644:errorcluster)  [unwired: 8 in, 1 out]
        "Write CSV File Error" <- w644
        n321 = case shown="Error .." w644 {
          tunnel: [TRUE ("File Saved\nWithout\nError") FALSE ("File Saved\nWithout\nError")] -> w647
          frame No Error {
          }
          frame Error {
          }
        }
      }
      frame 5 {
        # "write xml\nfile"
        # "convert\nto xml\nstring"
        # "Write config to File"
        n322 = Bundle By Name(cluster=T14 {"Write Config File Name"=path "", "Write Config File Comment"="", "WayPoints"=[], "TRAJECTORY_CONFIG"={"MaxVelocity"=0.0, "Max Acceleration"=0.0, "StartVelocity"=0.0, "End Velocity"=0.0, "Reversed"=FALSE, "DiffDrKineConstntDefined"=FALSE, "CentAcellConstntDefined"=FALSE, "DiffDrVoltConstntDefined"=FALSE, "DIFF_DRIVE_KINE_CONSTRAINT"={"Max Speed (M/S)"=0.0, "DIFF_DRIVE_KINEMATICS"={"TrackWidth_Meters"=0.0}, "Max Accel (M/S2)"=99999.0}, "CENTRIPETAL_ACCEL_CONSTRAINT"={"Max Cent Accel"=0.0}, "SwerveDrKineConstntDefined"=FALSE, "SWERVE_DRIVE_KINE_CONSTRAINT"={"Max Speed (M/S)"=0.0, "SwerveKinematics"={"NumModules"=0, "InverseKinematics"=[], "ForwardKinematics"=[], "Modules"=[], "PrevCoR"={"X"=0.0, "Y"=0.0}}}, "DIFF_DRIVE_VOLTAGE_CONSTRAINT"={"Max Voltage"=0.0, "DIFF_DRIVE_KINEMATICS"={"TrackWidth_Meters"=0.0}, "SIMPLE_MOTOR_FF"={"Ks"=0.0, "Kv"=0.0, "Ka"=0.0}}, "MECANUM_DRIVE_KINE_CONSTRAINT"={"Max Speed (M/S)"=0.0, "MECA_DRIVE_KINEMATICS"={"FrontLeft"={"X"=0.0, "Y"=0.0}, "FrontRight"={"X"=0.0, "Y"=0.0}, "RearLeft"={"X"=0.0, "Y"=0.0}, "RearRight"={"X"=0.0, "Y"=0.0}, "InverseKinematics"=[], "ForwardKinematics"=[], "PrevCoR"={"X"=0.0, "Y"=0.0}}}, "MecanumDrKineConstntDefined"=FALSE}, "IsCubic"=FALSE, "Units Selector"=enum."Inches", "UseWeights"=FALSE} ("TrajCreateConfig"), "Write Config File Name"="Write Config File Name", "Write Config File Comment"="Write Config File Comment", "WayPoints"=w789, "TRAJECTORY_CONFIG"=w788, "IsCubic"=w787, "Units Selector"=w778, "UseWeights"=w776) -> (w785:T14)
        n323 = local write "Trajectory File Comment"("Write Config File Comment") -> ()
        n324 = Flatten To XML(anything=w785) -> (xml string=w783:string)
        n325 = call-poly <vilib>:"Write to XML File.vi"("Standalone? (T)"=TRUE, "XML Input"=w783, "XML File Path"="Write Config File Name") -> ("error out"=w781:errorcluster)  [unwired: 6 in, 2 out]
        "Write Config FIle Error" <- w781
        n326 = case shown="No Error" w781 {
          tunnel: [TRUE ("File Saved\nWithout\nError") FALSE ("File Saved\nWithout\nError")] -> w780
          frame No Error {
          }
          frame Error {
          }
        }
      }
      frame 6 {
        # "End Program"
        n327 = disable-structure shown="Default" {
          frame condition #0 (active) {
            n328 = Stop() -> ()  [unwired: 1 in]
          }
          frame condition #1 {
            n329 = Quit LabVIEW() -> ()  [unwired: 1 in]
          }
        }
      }
    }
    "Trajectory\nCompleted\nError Free" <- w81
    "CSV File Saved\nWithout Error" <- w77
    "Config File Saved\nWithout Error" <- w30
    "JSON File Saved\nWithout Error" <- w15
  }
